vi "Eyecat_Omega_v01.vi"() -> ()   [LabVIEW 2014]
doc: "This VI is an upgrade from the WIN 1_v4 that implements the ageing subrutine"
uses:
  <vilib>/Utility/miscctls.llb/LVRowAndColumnTypeDef.ctl
  Buttons/Numeric control.ctl
  Buttons/String input.ctl
  Buttons/Numeric indicator.ctl
  Controls Win/Control 3.ctl
  <vilib>/Platform/TimedLoop/XDataNode/nitl_modes.ctl
  <vilib>/Platform/TimedLoop/XDataNode/timing_clust.ctl
  <vilib>/Platform/TimedLoop/XDataNode/wakeup.ctl
  <vilib>/Utility/miscctls.llb/LVComboBoxStrsAndValuesArrayTypeDef.ctl
  <vilib>/Utility/miscctls.llb/LVPositionTypeDef.ctl
  <vilib>/Utility/miscctls.llb/LVBoundsTypeDef.ctl
  <vilib>/Utility/file.llb/Read From Spreadsheet File (DBL).vi
  <vilib>/Utility/file.llb/Write To Spreadsheet File (string).vi
  <vilib>/Utility/file.llb/Read From Spreadsheet File (string).vi
  <vilib>/Platform/TimedLoop/XDataNode/XDataNode.xnode
  <vilib>/Platform/TimedLoop/XDataNode/XDNodeRunTimeDep.lvlib
panel:
  in  "Column Length":i32=12
  in  "Cycle Directory":string="c:\\Setup Files\\Ageing Cycles\\Omicron"
  in  "Omicron":bool
  out "Loop Number":dbl
  out "Mexa 3 IP":bool
  out "Mexa 2 IP":bool
  out "Mexa 1 IP":bool
  out "SMS":bool
  out "Directory":string
  out "Vehicle Name":string
  out "output cluster":T1
  out "SMS Recipients":u32
  out "Text Alerts":bool
  out "ETAS-D":bool
  out "ETAS Out":dbl[](array[numeric])
  out "MKS 1":dbl[](array[numeric])
  out "Mexa 3":dbl[](array[numeric])
  out "Mexa 2":dbl[](array[numeric])
  out "Mexa 1":dbl[](array[numeric])
  in  "Inlet LAMBDA Lean":T2=1.2 min=1.02 max=3.0 step=0.001
  in  "NO ppm SW":dbl=500.0 caption="NO (ppm)" min=0.0 max=500.0 step=1.0
  in  "Inlet Temperature (°C)":T2=400.0 min=350.0 max=1000.0 step=1.0
  out "File Directory":string
  out "OFF":bool
  out "COOL":bool
  out "TEST":bool
  out "WMUP":bool
  out "STBY":bool
  out "Mexa-3":bool
  out "Mexa-2":bool
  out "Mexa-1":bool
  out "Heat Load Control":bool
  out "Cycle Length":dbl
  out "Time Remaining":dbl=30.0 format="%<%H:%M:%S>t"
  out "Analysers":u32
  out "% Complete":u8(slide) scale=0.0..100.0
  out "Log?":bool
  in  "Total Number of Cycles":T2=1.0 min=1.0 max=10000.0 step=1.0
  in  "Sub-Cycle Pattern":string[][](table) caption="Subcycle pattern"
  in  "Delete Cycle":bool
  in  "Load Cycle":bool
  in  "Cycle Name":T3
  in  "Save Cycle":bool
  in  "Clear Cycle Pattern":bool
  in  "Menu_Tab":enum32{"Page 1"}(tab)
  in  "Back_Menu":bool
  in  "Home 2":bool
  in  "Performance 2":bool
  in  "Ageing 2":bool
  in  "System 2":bool
  in  "MFC 2":bool
  in  "Analyser 2":bool
  in  "Alarm 2":bool
  in  "Menu":bool
  out "MFC Array":dbl[](array[numeric])
  out "Valve Array":dbl[](array[numeric])
  out "MKS":bool
  out "Pressure":dbl
  out "ExtAnDn":bool
  out "ExtAnUp":bool
  out "File name":string
  out "Log interval (seconds)":T2
  in  "Flow rate Age":dbl
  in  "Inlet temp Age":dbl
  out "Stopped?":bool
  in  "Stop Cmd":T2
  out "Connected?":bool
  out "Error":dbl
  out "Iteration Duration":i64
  out "Finished Late? [i-1]":bool
  out "stop 2":bool
  in  "Enum 1":i16=1
  in  "Acknowledge":bool
  out "Test number":u16
  out "Flag1":bool=TRUE
  out "EditPos Subc":T4
  in  "Tab Control":T5(tab)
  in  "Admin":bool
  out "Warm Up":bool
  in  "Leak Test":bool
  in  "Stop Test":bool
  in  "Log Test Data":bool
  in  "Start Test":bool
  in  "Adv Settings":bool
  out "Doors Unlocked":bool
  in  "File Name":T3="Test"
  out "Fail":bool
  out "Pass":bool
  in  "Select Test Type":T6(radio)=enum."Ageing Test"
  out "Standby":bool
  out "Doors Open":bool
  out "Extractor Fan On":bool
  out "Test In Progress":bool
  out "Cool Down":bool
  out "System Alarm":bool
  in  "Nitrogen Injection (l/min)":T2=50.0 min=0.0 max=250.0 step=0.01
  in  "Oxidation Duration (min)":T2=1.0 min=0.0 max=60.0 step=0.01
  in  "Oxidation Wait (min)":T2=5.0 min=0.0 max=60.0 step=0.001
  in  "Reduction Duration (min)":T2=1.0 min=0.0 max=60.0 step=0.001
  in  "Reduction Wait (min)":T2=7.0 min=0.0 max=60.0 step=0.01
  out "OSC Results":string[][](table) caption="Subcycle pattern"
  in  "Test Stop temperature (°C)":T2=300.0 min=100.0 max=1000.0 step=1.0
  in  "Test Start Temperature (°C)":T2=125.0 min=0.0 max=500.0 step=1.0
  in  "Furnace Ramp Rate (°C/min)":T2=15.0 min=1.0 max=50.0 step=0.1
  in  "NO:CO Ratio":T2=1.1 min=1.0 max=5.0 step=0.1
  in  "Inlet O2 (%)":T2=0.5 min=0.0 max=14.0 step=0.01
  in  "Inlet LAMBDA":T2=1.0 min=0.6 max=3.0 step=0.001
  out "Space Velocity (h-1)":T7
  out "Vol Flow @ STP (l/min)":T7
  in  "Test Flow Rate(g/s)":T2 min=0.0 max=100.0 step=0.01
  out "Sample Volume (litres)":T7
  in  "Number of Samples":T2=1.0 min=1.0 max=6.0 step=1.0
  in  "Sample Diameter (mm)":T2
  out "CO Theory (%) NO":T7 format="%#_3g"
  out "CO Theory (%)":T7 format="%#_3g"
  out "HC Theory (%)":T7
  in  "Sample Length (mm)":T2 min=0.0 step=0.5
  in  "NO ppm Loff":T2 caption="NO ppm"
  in  "Ageing - Cycle Pattern":string[][](table) caption="Subcycle pattern"
  in  "Export Cycle":bool
  in  "Graph Cycle Box 2":string(combo)="CO"
  out "MFC Graph 6":dynamicdata(graph)
  in  "Graph Cycle Box":string(combo)="CO"
  in  "Compile Test Button 2":bool
  in  "Import Data":bool
  in  "Delete sCycle":bool
  in  "Save sCycle":bool
  in  "Load sCycle":bool
  in  "Clear subcycle":bool
  out "MFC Graph 5":dynamicdata(graph)
  out "Test Compiled":bool
  in  "Cycle List":i32(listbox)=1
  in  "Cycle Name":T3
  out "Heat Exchanger Temperatures (°C)":dynamicdata(graph)
  out "System Pressure (kPa)":dynamicdata(graph)
  out "Flow 2":dbl=30.0 format="%#.2g"
  out "Flow 1":dbl=30.0 format="%#.2g"
  out "TC 2":dbl=30.0 format="%#.3g"
  out "TC 6":dbl=30.0 format="%#.3g"
  out "TC 5":dbl=30.0 format="%#.3g"
  out "TC 4":dbl=30.0 format="%#.3g"
  out "TC 3":dbl=30.0 format="%#.3g"
  out "TC 1":dbl=30.0 format="%#.3g"
  out "Gas Flow Measurement Temperatures (°C)":dynamicdata(graph)
  out "Flow Rate (g/s)":dynamicdata(graph)
  out "Sample Temperatures (°C)":dynamicdata(graph)
  out "System Temperatures (°C)":dynamicdata(graph)
  in  "Graph 6 Box":string(combo)="NO"
  in  "Graph 5 Box":string(combo)="HC Cycle 1"
  out "MFC Graph 6":dynamicdata(graph)
  out "MFC Graph 5":dynamicdata(graph)
  in  "Graph 1 Box":string(combo)="CO"
  in  "Graph 4 Box":string(combo)="NO"
  in  "Graph 3 Box":string(combo)="Air Cycle 1"
  in  "Graph 2 Box":string(combo)="HC Cycle 1"
  out "MFC Graph 4":dynamicdata(graph)
  out "MFC Graph 3":dynamicdata(graph)
  out "MFC Graph 1":dynamicdata(graph)
  out "MFC Graph 2":dynamicdata(graph)
  out "CO2 Concentration (%)":dynamicdata(graph)
  out "Lambda":dynamicdata(graph)
  out "HC Concentration (ppm)":dynamicdata(graph)
  out "O2 Concentration (%)":dynamicdata(graph)
  out "CO Concentration (%)":dynamicdata(graph)
  out "NO Concentration (ppm)":dynamicdata(graph)
  in  "Purge System":bool
  in  "Alarm ack":bool
  in  "Clear log":bool
  out "Table":string[][](table)
  out "Soft Alarm":bool
  out "Hard Alarm":bool
  # "0.96 < lambda < 0.85"
  # "1.02< lambda < 1.6"
  # "350 < Tinlet < 1000"
  # "Test Commands"
  # "System Indicators"
  # "Test Type"
  # "Leak Test"
  # "Lightoff Settings"
  # "Catalyst Specification"
  # "Furnace Lightoff Settings"
  # "OSC Settings"
  # "CO/HC Lightoff Settings"
  # "Flow Specification"
  # "NO Lightoff Settings"
  # "Cycle Compiled"
  # "°C"
  # "°C"
  # "°C"
  # "°C"
  # "°C"
  # "°C"
  # "g/s"
  # "g/s"
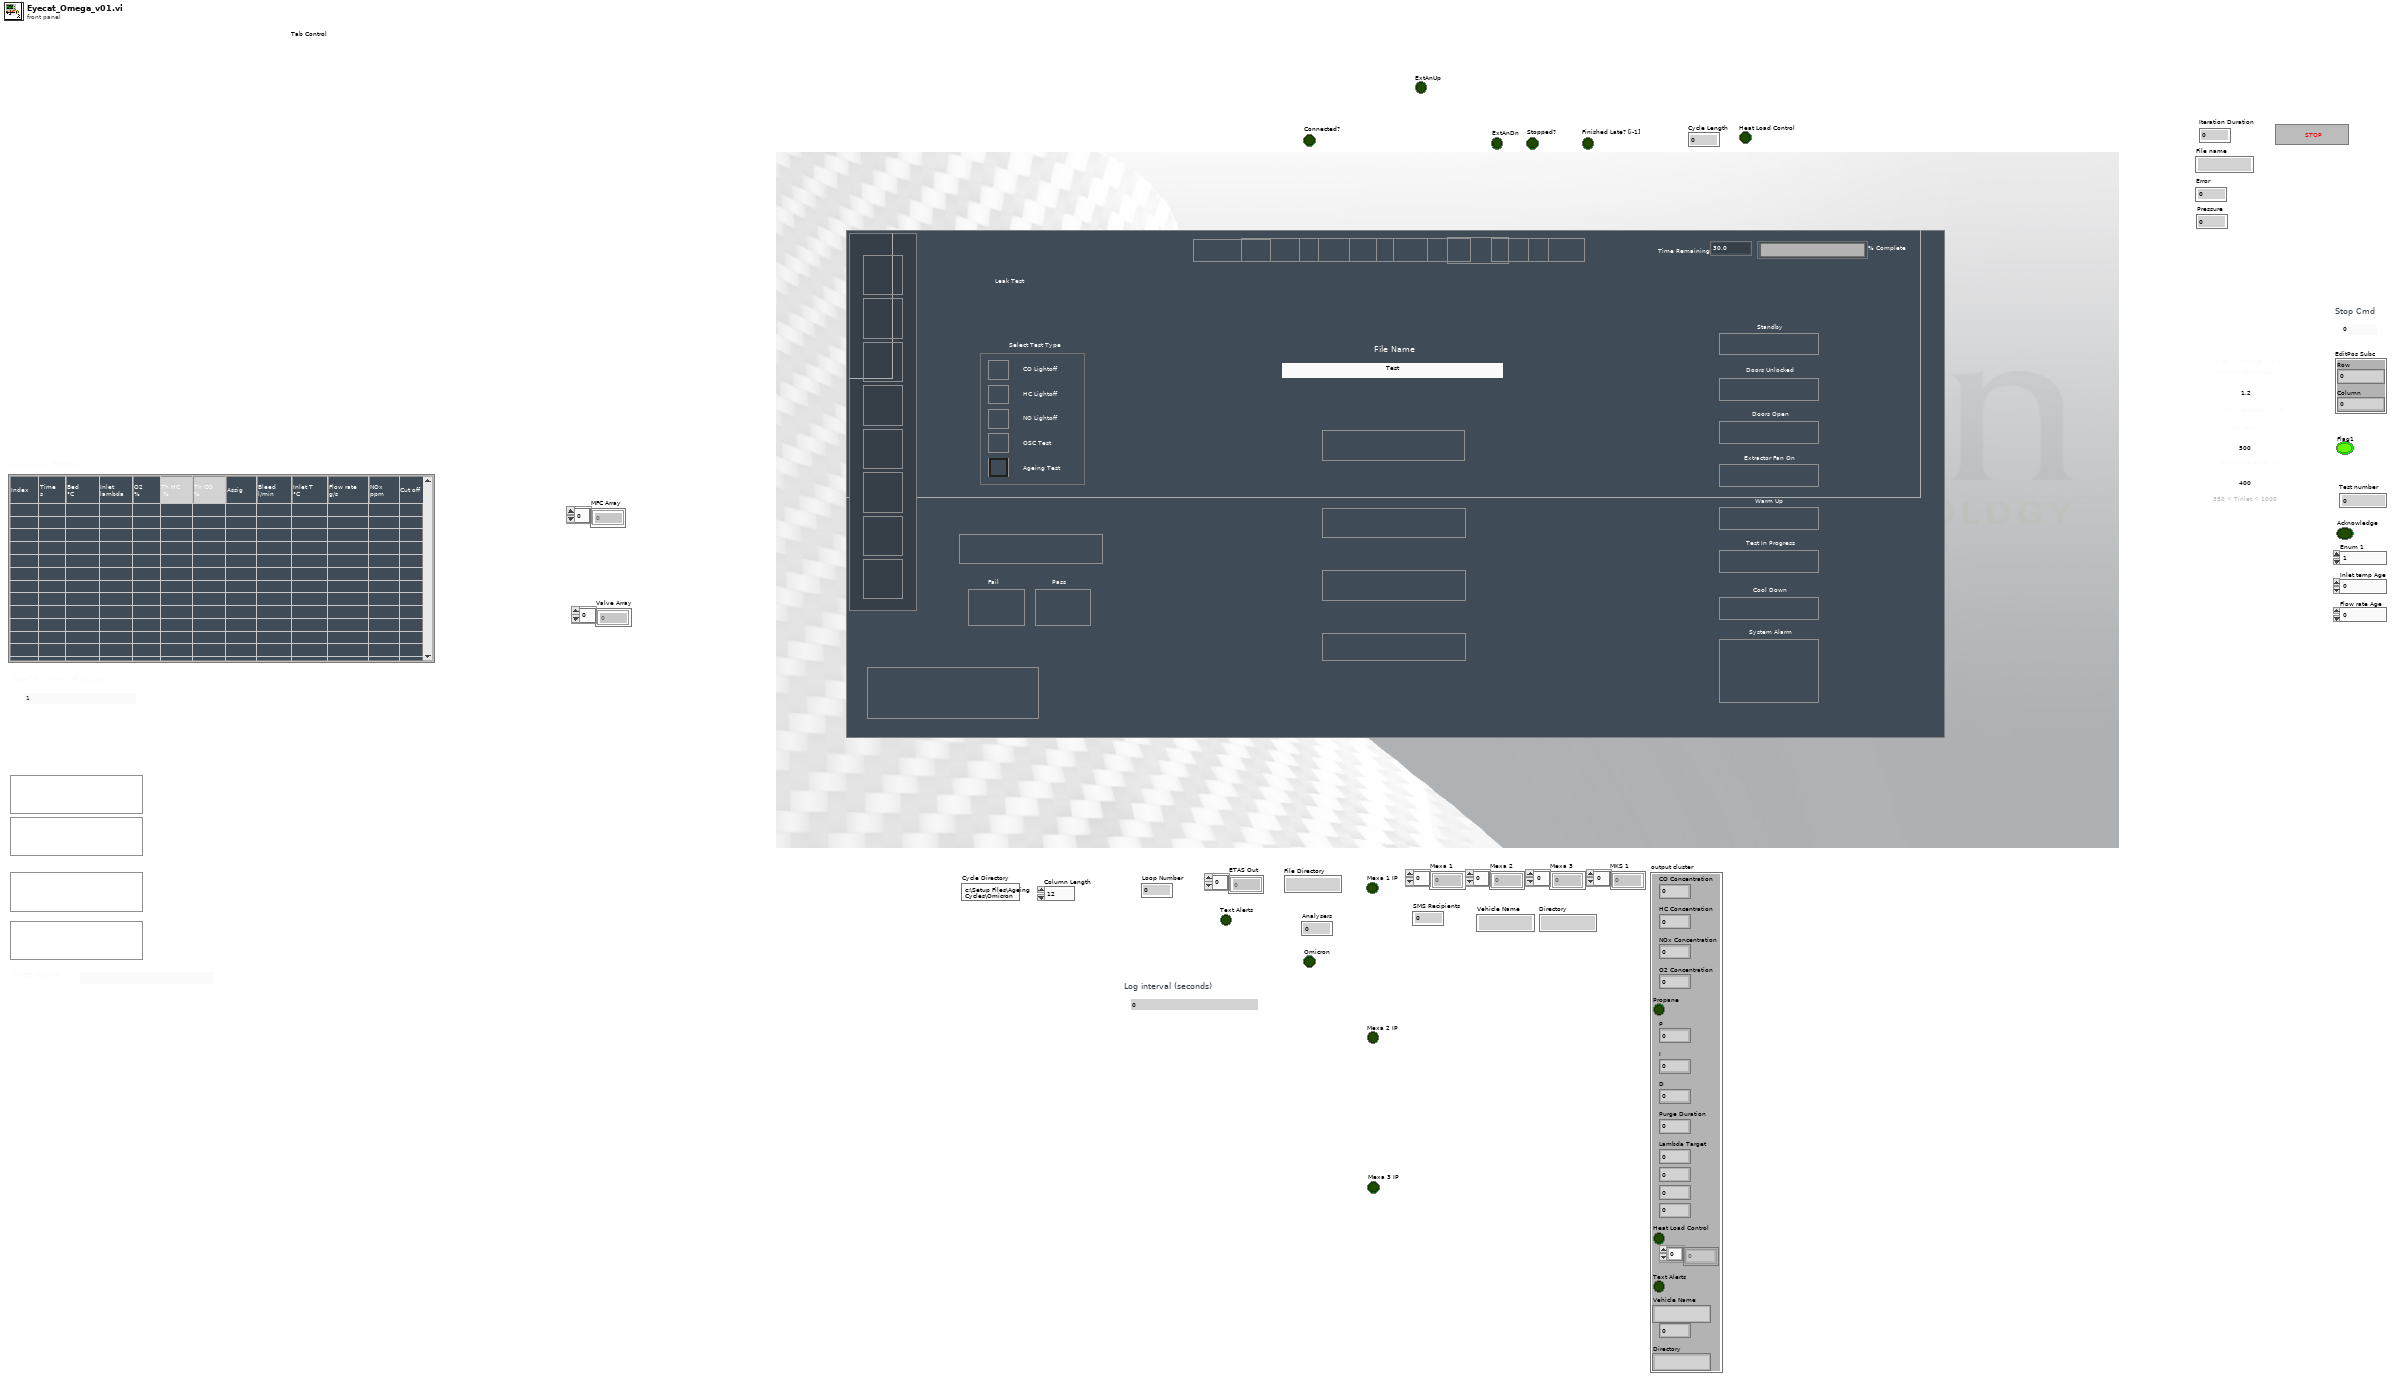
[diagram p1: front panel]
types:
  T1 = cluster{"CO Concentration":dbl, "HC Concentration":dbl, "NOx Concentration":dbl, "O2 Concentration":dbl, "Propane":bool, "P":dbl, "I":dbl, "D":dbl, "Purge Duration":dbl, "Lambda Target":dbl, dbl, u32, dbl, "Heat Load Control":bool, dbl[], "Text Alerts":bool, "Vehicle Name":string, u32, "Directory":string}
  T2 = typedef "Numeric control.ctl" = dbl
  T3 = typedef "String input.ctl" = string
  T4 = typedef "LVRowAndColumnTypeDef.ctl" = cluster{"Row":i32, "Column":i32}
  T5 = enum32{"MAIN", "PERFORMANCE TEST SETUP", "AGEING TEST SETUP", "SCHEDULE", "SYSTEM DATA", "MFC", "ANALYSER DATA", "ALARM LOG"}
  T6 = enum32{"CO Lightoff", "HC Lightoff", "NO Lightoff", "OSC Test", "Ageing Test"}
  T7 = typedef "Numeric indicator.ctl" = dbl
  T8 = typedef "XDNodeRunTimeDep.lvlib/nitl_modes.ctl" = enum32{"No Change", "Process missed periods, maintain original phase", "Discard missed periods, maintain original phase", "Process missed periods, ignore original phase", "Discard missed periods, ignore original phase"}
  T9 = typedef "Control 3.ctl" = enum16{"main", "start test", "save subc", "load subc", "delete subc", "clear table 1", "update list 1", "save cycle", "load cycle", "delete cycle", "clear table 2", "update list 2", "calc HC CO", "Total time calc", "update Cycle pattern ", "load cycle name", "convert to num", "load test array", "check scycle name", "check cycle name", "Multigas connect", "Multigas disconnect", "Leak Test", "Import Cycle", "Display Graph", "Export Cycle"}
  T10 = typedef "LVComboBoxStrsAndValuesArrayTypeDef.ctl" = cluster{"String":string, "Value":string}[]
  T11 = cluster{"CO Concentration":dbl, "CO Concentration":dbl, "CO Concentration":dbl, "CO Concentration":dbl, "Propane":bool, "CO Concentration":dbl, "CO Concentration":dbl, "CO Concentration":dbl, "CO Concentration":dbl, "CO Concentration":dbl, "CO Concentration":dbl, u32, "CO Concentration":dbl, "Propane":bool, dbl[], "Propane":bool, "Vehicle Name":string, u32, "Vehicle Name":string}
  T12 = typedef "XDNodeRunTimeDep.lvlib/timing_clust.ctl" = cluster{"Expected End [f-1]":u64, "Actual End [f-1]":u64, "Finished Late? [f-1]":bool, "Expected End [i-1]":u64, "Actual End [i-1]":u64, "Finished Late? [i-1]":bool, "Expected Start [i]":u64, "Actual Start [i]":u64, "Expected Start [f]":u64, "Actual Start [f]":u64, "Source Name":string, "Structure Name":string, "Period":i64, "Deadline":i64, "Offset":i64, "Start":i64, "Priority":i32, "Timeout":i32, "Mode":T8, "Wakeup Reason":T13, "Error":errorcluster, "Source Type":string, "Secondary Source Type":string, "Global End Time":u64, "Global Start Time":u64, "Frame Duration":u64, "Iteration Duration":u64, "Assigned CPU":i32, "I/O Scan Engine Mode":u32}
  T13 = typedef "XDNodeRunTimeDep.lvlib/wakeup.ctl" = enum32{"Normal", "Aborted", "Asynchronous wakeup", "Timing source error", "Timed loop error", "Timeout"}
  T14 = enum8{"Enabled", "Disabled", "Disabled and Grayed Out"}
  T15 = typedef "LVPositionTypeDef.ctl" = cluster{"Left":i32, "Top":i32}
  T16 = typedef "LVBoundsTypeDef.ctl" = cluster{"Width":u32, "Height":u32}
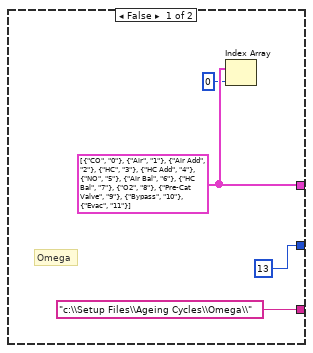
[diagram p2: hidden frame]
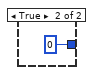
[diagram p4: hidden frame]
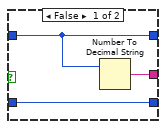
[diagram p5: hidden frame]
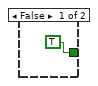
[diagram p7: hidden frame]
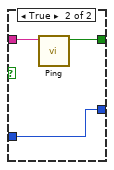
[diagram p9: hidden frame]
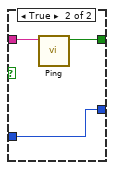
[diagram p11: hidden frame]
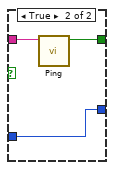
[diagram p13: hidden frame]
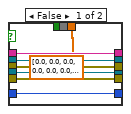
[diagram p15: hidden frame]
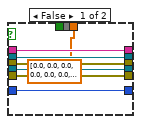
[diagram p16: hidden frame]
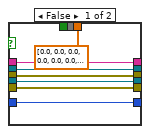
[diagram p17: hidden frame]
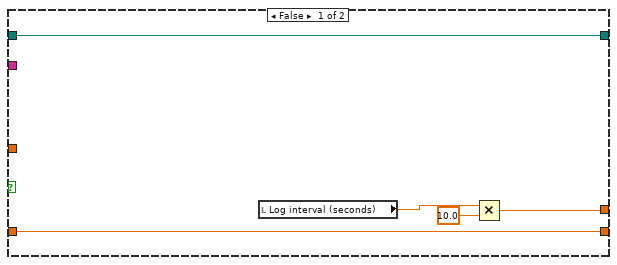
[diagram p18: hidden frame]
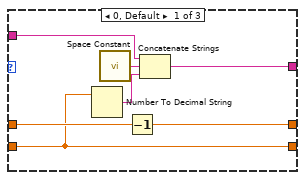
[diagram p19: hidden frame]
diagram:
  w1 = "6" ("Graph Cycle Box")
  w18 = u16 0 ("Test number")
  w40 = "" ("Vehicle Name")
  w39 = u32 0
  w41 = FALSE ("Propane")
  w42 = 0.0 ("CO Concentration")
  w44 = 0.0 ("Numeric")
  w30 = i64 50 ("Period")
  w13 = "C:\\Setup Files\\" ("string")
  (unwired) 12 ("length")
  w67 = FALSE ("Visible")
  w50 = i64 100 ("Period")
  w68 = FALSE
  w72 = FALSE
  w47 = 0.0 ("y")
  w84 = ""
  w89 = u32 13816530
  # "Menu Tabs"
  # "Initial Conditions"
  # "Ageing Table\nColumn No"
  # "0   Flow Rate 1\n1   Flow Rate 2\n     ECM 1\n     ECM 2\n2   CO2 U\n3   CO U\n4   HC U\n5   O2 U\n7   CO2 D\n8   CO D\n9   HC D\n10 O2 D\n12 TC1X\n13 TC2A\n14 TC3Y\n15 TC4B\n16 TC5\n17 TC6\n32 Venturi 1\n33 Venturi 2\n34 Tank\n35 Bearing 1\n36 Bearing 2\n38 Ex A\n39 Ex B\n40 Ex C\n41 Ex D\n     MFC Box\n42 Furnace 1\n43 Furnace 2\n44 NO 1 ?? \n45 Lambda 1\n46 NO 2 ??\n47 Lambda 2\n56 CO (L)\n57 CO (H)\n58CO2\n59 O2\n60 THC\n61 NO\n62 NOx\n63 NO2"
  # "~~~~~~~~~~~~~\n    Data Log Array\n~~~~~~~~~~~~~\n00 Status Integer\n01 Zero Constant\n\n02 DI no1 -errors\n03 DI no2 -states\n04 Flow rate 1 g/s\n05 Flow rate 2 g/s\n06 ECM 1 AFR\n07 ECM 2 AFR\n~~~~~~~~~~~~~\n     Mexa 518 - 1\n~~~~~~~~~~~~~\n08 CO2 %\n09 CO   %\n10 HC   ppm\n11 O2   %\n12 NOx ppm\n~~~~~~~~~~~~~\n     Mexa 518 - 2\n~~~~~~~~~~~~~\n13 CO2 %\n14 CO   %\n15 HC   ppm\n16 O2   %\n17 NOx ppm\n~~~~~~~~~~~~~\n     Temp Array I\n~~~~~~~~~~~~~\n18 1\n19 2 \n20 3\n21 4\n22 5\n23 6\n24 7\n25 8\n26 9\n27 10\n28 11\n29 12\n30 13\n31 14\n32 15\n33 16\n~~~~~~~~~~~~~\n     Temp Array II\n~~~~~~~~~~~~~\n34 17\n35 18\n36 19\n37 20\n38 Vent 1\n39 Vent 2\n40 Tank\n41 Bearing 1\n42 Bearing 2\n43 Cabinet\n44 Ex A\n45 Ex B\n46 Ex C\n47 Ex D\n48 Spare\n~~~~~~~~~~~~~\n49 Furnace Temp 1\n50 Furnace Temp 2\n51 Tank Pressure\n52 Rapidox\n~~~~~~~~~~~~~\n53 NOx L1\n54 NOx L2\n55 NOx 1\n56 NOx 2\n57 UEGO 1\n58 UEGO 2\n59 Switch Valve\n60 UEGO 3\n61 UEGO 4\n\n62 Teff\n\n63 Fan 1 Speed V\n64 Fan 2 Speed V"
  n1 = Concatenate Strings(w13, "Admin" ("string")) -> (w15:string)
  n2 = String To Path(string=w15) -> (path=w14:path)
  n3 = call-poly <vilib>:"Read From Spreadsheet File.vi"("file path (dialog if empty)"=w14) -> ("first row"=w9:dbl[])  [unwired: 6 in, 4 out]
  n4 = Index Array(array=w9, index=15) -> (element=w10:dbl)
  n5 = Number To Boolean Array(number=w10) -> (Boolean array=w12:bool[])
  n6 = Index Array(array=w12, index=2) -> (element=w7:bool)
  n7 = case shown="True" w7 {
    tunnel: ["c:\\Setup Files\\Ageing Cycles\\Omega\\" "c:\\Setup Files\\Ageing Cycles\\Omicron\\"] -> w5
    tunnel: [13 ("length") 20 ("length")] -> w2
    tunnel: [w96 T10 [{"String"="CO-1", "Value"="0"}, {"String"="Air-1", "Value"="1"}, {"String"="Air-1 Add", "Value"="2"}, {"String"="HC-1", "Value"="3"}, {"String"="HC-1 Add", "Value"="4"}, {"String"="O2-1", "Value"="5"}, {"String"="CO-2", "Value"="6"}, {"String"="Air-2", "Value"="7"}, {"String"="Air-2 Add", "Value"="8"}, {"String"="HC-2", "Value"="9"}, {"String"="HC-2 Add", "Value"="10"}, {"String"="O2-2", "Value"="11"}, {"String"="Air Bal", "Value"="12"}, {"String"="HC Bal", "Value"="13"}, {"String"="Cat-1 Valve", "Value"="14"}, {"String"="Cat-2 Valve", "Value"="15"}, {"String"="Bypass Valve", "Value"="16"}, {"String"="Evac-1", "Value"="17"}, {"String"="Evac-2", "Value"="18"}] ("Strings And Values []")] -> w4
    frame False {
      w96 = T10 [{"String"="CO", "Value"="0"}, {"String"="Air", "Value"="1"}, {"String"="Air Add", "Value"="2"}, {"String"="HC", "Value"="3"}, {"String"="HC Add", "Value"="4"}, {"String"="NO", "Value"="5"}, {"String"="Air Bal", "Value"="6"}, {"String"="HC Bal", "Value"="7"}, {"String"="O2", "Value"="8"}, {"String"="Pre-Cat Valve", "Value"="9"}, {"String"="Bypass", "Value"="10"}, {"String"="Evac", "Value"="11"}] ("Strings And Values []")
      # "Omega"
      n8 = Index Array(array=w96, index=0) -> ()  [unwired: 1 out]
    }
    frame True {
      # "Omicron"
    }
  }
  n9 = local write "Cycle Name"(w84) -> ()
  n10 = local write "Cycle Name"(w84) -> ()
  n11 = local write "Test Compiled"(FALSE ("Cycle Compiled")) -> ()
  n12 = local write "Flag1"(FALSE) -> ()
  n13 = local write "Analysers"(u32 0 ("Analysers")) -> ()
  n14 = local write "Sub-Cycle Pattern"(string[][] [["", "0", "", "", "", "", "", "", "", "", "", "", ""], ["", "", "", "", "", "", "", "", "", "", "", "", ""], ["", "", "", "", "", "", "", "", "", "", "", "", ""], ["", "", "", "", "", "", "", "", "", "", "", "", ""], ["", "", "", "", "", "", "", "", "", "", "", "", ""], ["", "", "", "", "", "", "", "", "", "", "", "", ""], ["", "", "", "", "", "", "", "", "", "", "", "", ""], ["", "", "", "", "", "", "", "", "", "", "", "", ""], ["", "", "", "", "", "", "", "", "", "", "", "", ""], ["", "", "", "", "", "", "", "", "", "", "", "", ""], ["", "", "", "", "", "", "", "", "", "", "", "", ""], ["", "", "", "", "", "", "", "", "", "", "", "", ""], ["", "", "", "", "", "", "", "", "", "", "", "", ""], ["", "", "", "", "", "", "", "", "", "", "", "", ""], ["", "", "", "", "", "", "", "", "", "", "", "", ""], ["", "", "", "", "", "", "", "", "", "", "", "", ""], ["", "", "", "", "", "", "", "", "", "", "", "", ""], ["", "", "", "", "", "", "", "", "", "", "", "", ""], ["", "", "", "", "", "", "", "", "", "", "", "", ""], ["", "", "", "", "", "", "", "", "", "", "", "", ""], ["", "", "", "", "", "", "", "", "", "", "", "", ""], ["", "", "", "", "", "", "", "", "", "", "", "", ""], ["", "", "", "", "", "", "", "", "", "", "", "", ""], ["", "", "", "", "", "", "", "", "", "", "", "", ""], ["", "", "", "", "", "", "", "", "", "", "", "", ""], ["", "", "", "", "", "", "", "", "", "", "", "", ""], ["", "", "", "", "", "", "", "", "", "", "", "", ""], ["", "", "", "", "", "", "", "", "", "", "", "", ""], ["", "", "", "", "", "", "", "", "", "", "", "", ""], ["", "", "", "", "", "", "", "", "", "", "", "", ""], ["", "", "", "", "", "", "", "", "", "", "", "", ""]]) -> ()
  n15 = shared-variable "RT CompactRIO Target\\Library 1.lvlib\\Enum 1"(u16 0 ("Enum 1")) -> ()  [unwired: 1 in, 1 out]
  n16 = property on="Tab Control" class="TabCtl (strict)"("Value"=T5."MAIN" ("Tab Control")) -> ()  [unwired: 2 in, 2 out]
  n17 = Bundle("CO Concentration"=w42, "CO Concentration"=w42, "CO Concentration"=w42, "CO Concentration"=w42, "Propane"=w41, "CO Concentration"=w42, "CO Concentration"=w42, "CO Concentration"=w42, "CO Concentration"=w42, "CO Concentration"=w42, "CO Concentration"=w42, w39, "CO Concentration"=w42, "Propane"=w41, dbl[] [0.0, 0.0, 0.0, 2.0, 1.0], "Propane"=w41, "Vehicle Name"=w40, w39, "Vehicle Name"=w40) -> (w43:T11)  [unwired: 1 in]
  n18 = local write "output cluster"(w43) -> ()
  n19 = property on="Sub-Cycle Pattern" class="Tbl (strict)"("Active Cell"=T4 {"Row"=-2, "Column"=5} ("Active Cell:Active Cell"), "Cell BG Color"=w89) -> (error out=w90:errorcluster)  [unwired: 2 in, 1 out]
  n20 = property on="Sub-Cycle Pattern" class="Tbl (strict)"(error in=w90, "Active Cell"=T4 {"Row"=-2, "Column"=6} ("Active Cell:Active Cell"), "Cell BG Color"=w89) -> ()  [unwired: 1 in, 2 out]
  n21 = local write "Fail"(w72) -> ()
  n22 = local write "Pass"(w72) -> ()
  n23 = property on="Pass" class="Bool (strict)"("Value"=w72) -> ()  [unwired: 2 in, 2 out]
  n24 = property on="Fail" class="Bool (strict)"("Value"=w72) -> ()  [unwired: 2 in, 2 out]
  n25 = property on="System Alarm" class="Bool (strict)"("Value"=w72) -> ()  [unwired: 2 in, 2 out]
  n26 = property on="Soft Alarm" class="Bool (strict)"("Value"=w72) -> ()  [unwired: 2 in, 2 out]
  n27 = property on="Hard Alarm" class="Bool (strict)"("Value"=w72) -> ()  [unwired: 2 in, 2 out]
  n28 = property on="TEST" class="Bool (strict)"("Visible"=w67) -> ()  [unwired: 2 in, 2 out]
  n29 = property on="OFF" class="Bool (strict)"("Visible"=w67) -> ()  [unwired: 2 in, 2 out]
  n30 = property on="WMUP" class="Bool (strict)"("Visible"=w67) -> ()  [unwired: 2 in, 2 out]
  n31 = property on="STBY" class="Bool (strict)"("Visible"=w67) -> ()  [unwired: 2 in, 2 out]
  n32 = property on="COOL" class="Bool (strict)"("Visible"=w67) -> ()  [unwired: 2 in, 2 out]
  n33 = local write "Connected?"(w72) -> ()
  n34 = local write "Acknowledge"(w72) -> ()
  n35 = String To Path(string="c:\\Setup Files\\Cycles Folder\\") -> (path=w86:path)
  n36 = String To Path(string=w5) -> (path=w87:path)
  n37 = List Folder(path=w86, pattern="*.eyec") -> ()  [unwired: 2 in, 4 out]
  n38 = List Folder(path=w87, pattern="*.eyes") -> (filenames=w88:string[])  [unwired: 2 in, 3 out]
  n39 = Obtain Queue(element data type=Control_3."main" ("Enum")) -> (queue out=w93:refnum<queue>)  [unwired: 4 in, 2 out]
  n40 = property on="Cycle Directory" class="Str"("Value"=w5) -> ()  [unwired: 2 in, 2 out]
  n41 = Decrement(x=w2) -> (x-1=w3:i32)
  n42 = property on="Graph Cycle Box" class="CmbBox"("Strings And Values[]"=w4, "Value"=w1) -> ()  [unwired: 2 in, 2 out]
  n43 = property on="Graph Cycle Box 2" class="CmbBox"("Strings And Values[]"=w4, "Value"=w1) -> ()  [unwired: 2 in, 2 out]
  n44 = property on="Cycle List" class="LstBox (strict)"("Item Names"=w88) -> ()  [unwired: 2 in, 2 out]
  n45 = local write "Mexa 1 IP"(FALSE ("Mexa 1 IP")) -> ()
  n46 = property on="Column Length" class="DigNum (strict)"("Value"=w3) -> ()  [unwired: 2 in, 2 out]
  n47 = Concatenate Strings(w13, "Admin" ("string")) -> (w64:string)
  n48 = Concatenate Strings(w13, "Admin IP" ("string")) -> (w63:string)
  n49 = String To Path(string=w63) -> (path=w31:path)
  n50 = String To Path(string=w64) -> (path=w61:path)
  n51 = node-c288(w50) -> (w60:T12)  [unwired: 3 in]
  n52 = node-c288(w50) -> (w58:T12)  [unwired: 3 in]
  n53 = node-c288(w50) -> (w56:T12)  [unwired: 3 in]
  n54 = node-c288() -> (w54:T12)  [unwired: 4 in]
  n55 = node-c288(w50) -> (w52:T12)  [unwired: 3 in]
  n56 = timed-loop {
    timing: w60 -> [_]
    timing-out: [_] -> w59
    shift-right: [w116] -> _
    shift-left: _ -> [w115]
    shift-right: [w113] -> _
    shift-left: _ -> [w109]
    shift-right: [w114] -> _
    shift-left: _ -> [w110]
    shift-right: [w112] -> _
    shift-left: _ -> [w108]
    shift-right: [w111] -> _
    shift-left: _ -> [w107]
    shift-right: [w106] -> _
    shift-left: _ -> [w105]
    tunnel: w31 -> [w103]
    stop <- _ stop-if-true
    n57 = node-c288() -> ()  [unwired: 1 in, 1 out]
    n58 = call-poly <vilib>:"Read From Spreadsheet File.vi"("file path (dialog if empty)"=w103) -> ("first row"=w123:string[])  [unwired: 6 in, 4 out]
    n59 = local read "Analysers"() -> (w120:u32)
    n60 = Array Subset(array=w123, index=0 ("length"), length=2) -> (w121:string[])
    n61 = Number To Boolean Array(number=w120) -> (Boolean array=w119:bool[])
    n62 = local read "Mexa 1 IP"() -> (w102:bool)
    n63 = Index Array(array=w119, index=0) -> (element=w117:bool)
    "Mexa-1" <- w117
    n64 = case shown="True" w102 {
      tunnel: w121 -> [_ w146]
      tunnel: w117 -> [_ w145]
      tunnel: [w131 w144] -> w116
      tunnel: w115 -> [w131 w143]
      tunnel: [w130 w142] -> w114
      tunnel: [w129 w141] -> w113
      tunnel: [w128 w140] -> w112
      tunnel: [w127 w139] -> w111
      tunnel: w110 -> [w130 w138]
      tunnel: w109 -> [w129 w137]
      tunnel: w108 -> [w128 w136]
      tunnel: w107 -> [w127 w135]
      tunnel: [w126 w134] -> w106
      tunnel: w105 -> [w126 w133]
      tunnel: [dbl[] [0.0, 0.0, 0.0, 0.0, 0.0, 0.0, 0.0] ("Emissions") w132] -> w104
      frame False {
      }
      frame True {
        n65 = call "Mexa_7170.vi"("String 1 In"=w143, "Connect"=w145, "IP Array"=w146, "connection ID 1 In"=w138, "error out 1 In"=w137, "connection ID 2 In"=w136, "error out 2 In"=w135, "Time In"=w133) -> ("Emissions"=w132:dbl[], "String 1 Out"=w144:string, "connection ID 1 Out"=w142:refnum<k5>, "error 1 out"=w141:errorcluster, "connection ID 2 Out"=w140:refnum<k16>, "Time Out"=w134:i16, "error 2 out"=w139:errorcluster)  [unwired: 1 in]
      }
    }
    "Mexa 1" <- w104
    n66 = node-c288() -> ()  [unwired: 1 in, 1 out]
  }
  n67 = timed-loop {
    timing: w58 -> [_]
    timing-out: [_] -> w57
    shift-right: [w163] -> _
    shift-left: _ -> [w164]
    shift-right: [w161] -> _
    shift-left: _ -> [w157]
    shift-right: [w162] -> _
    shift-left: _ -> [w158]
    shift-right: [w160] -> _
    shift-left: _ -> [w156]
    shift-right: [w159] -> _
    shift-left: _ -> [w155]
    shift-right: [w153] -> _
    shift-left: _ -> [w154]
    tunnel: w31 -> [w166]
    stop <- _ stop-if-true
    n68 = node-c288() -> ()  [unwired: 1 in, 1 out]
    n69 = call-poly <vilib>:"Read From Spreadsheet File.vi"("file path (dialog if empty)"=w166) -> ("first row"=w171:string[])  [unwired: 6 in, 4 out]
    n70 = local read "Analysers"() -> (w169:u32)
    n71 = Array Subset(array=w171, index=2 ("length"), length=2) -> (w165:string[])
    n72 = Number To Boolean Array(number=w169) -> (Boolean array=w168:bool[])
    n73 = local read "Mexa 2 IP"() -> (w149:bool)
    n74 = Index Array(array=w168, index=1) -> (element=w152:bool)
    "Mexa-2" <- w152
    n75 = case shown="True" w149 {
      tunnel: w165 -> [_ w194]
      tunnel: w164 -> [w179 w193]
      tunnel: [w179 w192] -> w163
      tunnel: [w178 w191] -> w162
      tunnel: [w177 w190] -> w161
      tunnel: [w176 w189] -> w160
      tunnel: [w175 w188] -> w159
      tunnel: w158 -> [w178 w187]
      tunnel: w157 -> [w177 w186]
      tunnel: w156 -> [w176 w185]
      tunnel: w155 -> [w175 w184]
      tunnel: w154 -> [w174 w183]
      tunnel: [w174 w182] -> w153
      tunnel: w152 -> [_ w181]
      tunnel: [dbl[] [0.0, 0.0, 0.0, 0.0, 0.0, 0.0, 0.0] ("Emissions") w180] -> w151
      frame False {
      }
      frame True {
        n76 = call "Mexa_7170 - 2.vi"("String 1 In"=w193, "Connect"=w181, "IP Array"=w194, "connection ID 1 In"=w187, "error out 1 In"=w186, "connection ID 2 In"=w185, "error out 2 In"=w184, "Time In"=w183) -> ("Emissions"=w180:dbl[], "String 1 Out"=w192:string, "connection ID 1 Out"=w191:refnum<k5>, "error 1 out"=w190:errorcluster, "connection ID 2 Out"=w189:refnum<k16>, "Time Out"=w182:i16, "error 2 out"=w188:errorcluster)  [unwired: 1 in]
      }
    }
    n77 = call "7000string to array.vi"("7170 Input"=w151) -> ("7000 Out"=→"Mexa 2":dbl[])  [unwired: 4 in]
    n78 = node-c288() -> ()  [unwired: 1 in, 1 out]
  }
  n79 = timed-loop {
    timing: w56 -> [_]
    timing-out: [_] -> w55
    shift-right: [w211] -> _
    shift-left: _ -> [w212]
    shift-right: [w207] -> _
    shift-left: _ -> [w204]
    shift-right: [w210] -> _
    shift-left: _ -> [w205]
    shift-right: [w209] -> _
    shift-left: _ -> [w203]
    shift-right: [w208] -> _
    shift-left: _ -> [w202]
    shift-right: [w206] -> _
    shift-left: _ -> [w201]
    tunnel: w31 -> [w214]
    stop <- _ stop-if-true
    n80 = node-c288() -> ()  [unwired: 1 in, 1 out]
    n81 = call-poly <vilib>:"Read From Spreadsheet File.vi"("file path (dialog if empty)"=w214) -> ("first row"=w219:string[])  [unwired: 6 in, 4 out]
    n82 = local read "Analysers"() -> (w217:u32)
    n83 = Array Subset(array=w219, index=4 ("length"), length=2) -> (w199:string[])
    n84 = Number To Boolean Array(number=w217) -> (Boolean array=w216:bool[])
    n85 = local read "Mexa 3 IP"() -> (w197:bool)
    n86 = Index Array(array=w216, index=2) -> (element=w200:bool)
    "Mexa-3" <- w200
    n87 = case shown="True" w197 {
      tunnel: w212 -> [w227 w242]
      tunnel: [w227 w241] -> w211
      tunnel: [w226 w240] -> w210
      tunnel: [w224 w239] -> w209
      tunnel: [w223 w238] -> w208
      tunnel: [w225 w237] -> w207
      tunnel: [w222 w236] -> w206
      tunnel: w205 -> [w226 w235]
      tunnel: w204 -> [w225 w234]
      tunnel: w203 -> [w224 w233]
      tunnel: w202 -> [w223 w232]
      tunnel: w201 -> [w222 w231]
      tunnel: w200 -> [_ w230]
      tunnel: w199 -> [_ w229]
      tunnel: [dbl[] [0.0, 0.0, 0.0, 0.0, 0.0, 0.0, 0.0] ("Emissions") w228] -> w198
      frame False {
      }
      frame True {
        n88 = call "Mexa_7170 - 3.vi"("String 1 In"=w242, "Connect"=w230, "IP Array"=w229, "connection ID 1 In"=w235, "error out 1 In"=w234, "connection ID 2 In"=w233, "error out 2 In"=w232, "Time In"=w231) -> ("Emissions"=w228:dbl[], "String 1 Out"=w241:string, "connection ID 1 Out"=w240:refnum<k5>, "error 1 out"=w237:errorcluster, "connection ID 2 Out"=w239:refnum<k16>, "Time Out"=w236:i16, "error 2 out"=w238:errorcluster)  [unwired: 1 in]
      }
    }
    n89 = call "7000string to array.vi"("7170 Input"=w198) -> ("7000 Out"=→"Mexa 3":dbl[])  [unwired: 4 in]
    n90 = node-c288() -> ()  [unwired: 1 in, 1 out]
  }
  n91 = timed-loop {
    timing: w54 -> [_]
    timing-out: [_] -> w53
    tunnel: w31 -> [w248]
    stop <- _ stop-if-true
    n92 = node-c288() -> ()  [unwired: 1 in, 1 out]
    n93 = call-poly <vilib>:"Read From Spreadsheet File.vi"("file path (dialog if empty)"=w248) -> ("first row"=w253:string[])  [unwired: 6 in, 4 out]
    n94 = local read "Analysers"() -> (w251:u32)
    n95 = Array Subset(array=w253, index=6 ("length"), length=2) -> (w247:string[])
    n96 = Number To Boolean Array(number=w251) -> (Boolean array=w250:bool[])
    n97 = Index Array(array=w250, index=3) -> (element=w246:bool)
    "MKS" <- w246
    n98 = call "MKS.vi"("IP Array"=w247, "Connect"=w246) -> ("Emissions"=→"MKS 1":dbl[])  [unwired: 9 in]
    n99 = node-c288() -> ()  [unwired: 1 in, 1 out]
  }
  n100 = timed-loop {
    timing: w52 -> [_]
    timing-out: [_] -> w51
    tunnel: w31 -> [w275]
    shift-right: [w274] -> _
    shift-left: _ -> [w270]
    shift-right: [w273] -> _
    shift-left: _ -> [w269]
    shift-right: [w272] -> _
    shift-left: _ -> [w268]
    shift-right: [w271] -> _
    shift-left: _ -> [w267]
    shift-right: [w259] -> _
    shift-left: _ -> [w257]
    stop <- _ stop-if-true
    n101 = node-c288() -> ()  [unwired: 1 in, 1 out]
    n102 = call-poly <vilib>:"Read From Spreadsheet File.vi"("file path (dialog if empty)"=w275) -> ("first row"=w280:string[])  [unwired: 6 in, 4 out]
    n103 = local read "Analysers"() -> (w278:u32)
    n104 = Number To Boolean Array(number=w278) -> (Boolean array=w277:bool[])
    n105 = Index Array(array=w280, index=8 ("length")) -> (element=w261:string)
    n106 = Index Array(array=w277, index=4) -> (element=w260:bool)
    "ETAS-D" <- w260
    n107 = call "ETAS_Driver_1.0.2.vi"("Counter In"=w267, "IP Address"=w261, "Loop In"=w268, "error In"=w269, "Reference In"=w270, "Etas Connect"=w260) -> ("Loop Out"=w272:i32, "error out"=w273:errorcluster, "Reference Out"=w274:refnum<k24>, "ETAS Out"=w258:dbl[], "Counter Out"=w271:dbl)  [unwired: 1 in]
    n108 = Index Array(array=w258) -> (element #1=w264:dbl, element #2=w263:dbl)  [unwired: 2 in]
    n109 = Equal To 0?(x=w264) -> (x = 0?=w266:bool)
    n110 = Equal To 0?(x=w263) -> (x = 0?=w265:bool)
    n111 = Compound Arithmetic op=AND(w266, w265, w260) -> (w262:bool)
    n112 = case shown="True" w262 {
      tunnel: [w281 w282] -> w259
      tunnel: w257 -> [_ w282]
      tunnel: w258 -> [w281 _]
      frame False {
      }
      frame True {
      }
    }
    "ETAS Out" <- w259
    n113 = node-c288() -> ()  [unwired: 1 in, 1 out]
  }
  n114 = while {
    tunnel: w93 -> [w292]
    tunnel: [FALSE ("stop 2")] -> w78
    tunnel: w61 -> [w289]
    stop <- w293 stop-if-true
    n115 = Concatenate Strings("Cycle Directory", "\\" ("string")) -> (w285:string)
    n116 = Dequeue Element(queue=w292) -> (element=w291:T9)  [unwired: 2 in, 3 out]
    n117 = case shown="\"load test array\"" w291 {
      tunnel: w285 -> [_ _ _ w351 w362 w399 w432 w463 _ _ _ _ _ _ _ _ _ _ _ _ _ _ _ _ _ w729]
      tunnel: w289 -> [w310 _ _ _ _ _ _ _ _ _ _ _ _ _ _ _ _ w529 _ _ _ _ _ _ _ _]
      tunnel: "Column Length" -> [_ _ _ _ _ w396 w431 _ _ _ _ _ _ _ _ _ _ w536 _ _ _ _ _ _ _ w718]
      frame "main", Default {
        w308 = 600.0 ("y")
        # "Advanced Settings"
        # "OSC Inputs"
        # "35"
        # "0"
        # "Output Cluster\n\n0 CO Conc %\n1 HC Conc %\n2 NOx Conc %\n3 O2 Conc %\n4 Propane/Propylene\n5 lambda P\n6 lambda I\n7 lambda D\n8 purge duration\n9 Target furnace lambda\n10 Log Interval\n11 Analysers\n12 Cycle Length\n13 Heat Load Control\n14 Ref Temp\n15 C Factor\n16 Target Heat Load\n17 Control TC 1\n18 Control TC 2"
        # "00 stop cmd\n01 Test Number\n02 Test Flow Rate\n03 Test Start Temperature\n04 Test Stop Temperature\n05 Furnace Ramp Rate\n06 Inlet Lambda\n07 Inlet O2\n08 Inlet Lambda Rich\n09 Inlet Lambda Lean\n10 Inlet Temperature\n11 NO SW"
        # "20"
        # "25"
        # "30"
        # "10"
        # "5"
        # "0"
        # "25"
        # "20"
        # "15"
        # "10"
        # "5"
        n118 = call-poly <vilib>:"Read From Spreadsheet File.vi"("file path (dialog if empty)"=w310) -> ("first row"=w309:dbl[])  [unwired: 6 in, 4 out]
        n119 = local read "output cluster"() -> (w329:T1)
        n120 = Multiply(x="Oxidation Duration (min)", y=w308) -> (x*y=w303:T2)
        n121 = Multiply(x="Oxidation Wait (min)", y=w308) -> (x*y=w302:T2)
        n122 = Multiply(x="Reduction Duration (min)", y=w308) -> (x*y=w301:T2)
        n123 = Multiply(x="Reduction Wait (min)", y=w308) -> (x*y=w300:T2)
        n124 = local read "Test number"() -> (w342:u16)
        n125 = Unbundle(w329) -> ("CO Concentration"=w322:dbl, "HC Concentration"=w321:dbl, "NOx Concentration"=w320:dbl, "O2 Concentration"=w319:dbl, "Propane"=w317:bool, "P"=w326:dbl, "I"=w325:dbl, "D"=w324:dbl, "Purge Duration"=w327:dbl, "Lambda Target"=w328:dbl, →"Log interval (seconds)":dbl, →"Analysers":u32, w313:dbl, "Heat Load Control"=w315:bool, w311:dbl[], "Text Alerts"=→"Text Alerts":bool, "Vehicle Name"=→"Vehicle Name":string, →"SMS Recipients":u32, "Directory"=→"Directory":string)
        "Cycle Length" <- w313
        "Heat Load Control" <- w315
        n126 = local read "HC Theory (%)"() -> (w318:T7)
        n127 = Boolean To (0,1)(Boolean=w317) -> (0, 1=w316:i16)
        n128 = Boolean To (0,1)(Boolean=w315) -> (0, 1=w312:i16)
        n129 = local read "Test Flow Rate(g/s)"() -> (w337:T2)
        n130 = local read "NO ppm Loff"() -> (w330:T2)
        n131 = local read "CO Theory (%)"() -> (w331:T7)
        n132 = local read "Inlet O2 (%)"() -> (w332:T2)
        n133 = Build Array (concatenate)("Stop Cmd", w342, w337, "Test Start Temperature (°C)", "Test Stop temperature (°C)", "Furnace Ramp Rate (°C/min)", w332, w331, w318, "Inlet LAMBDA Lean", "Inlet Temperature (°C)", "NO ppm SW", w330, "Nitrogen Injection (l/min)", w303, w302, w301, w300, w322, w321, w320, w319, w316, w326, w325, w324, w327, w328, w313, w312, w311, w309) -> (w334:T2[])
        n134 = shared-variable "RT CompactRIO Target\\Library 1.lvlib\\Control Variables"(w334) -> ()  [unwired: 1 in, 1 out]
        "Test number" <- "Select Test Type"
      }
      frame "start test" {
        w343 = FALSE
        n135 = property on="Pass" class="Bool (strict)"("Value"=w343) -> ()  [unwired: 2 in, 2 out]
        n136 = property on="Fail" class="Bool (strict)"("Value"=w343) -> ()  [unwired: 2 in, 2 out]
        n137 = local write "Pass"(w343) -> ()
        n138 = local write "Fail"(w343) -> ()
        n139 = shared-variable "RT CompactRIO Target\\Library 1.lvlib\\Enum 1"("Enum 1") -> ()  [unwired: 1 in, 1 out]
      }
      frame "clear table 1" {
        n140 = property on="Sub-Cycle Name" class="Str (strict)"("Value"="" ("Subcycle name")) -> ()  [unwired: 2 in, 2 out]
        n141 = local write "Ageing - Cycle Pattern"(string[][] [["", "0", "", "", "", "", "", "", "", "", "", "", ""], ["", "", "", "", "", "", "", "", "", "", "", "", ""], ["", "", "", "", "", "", "", "", "", "", "", "", ""], ["", "", "", "", "", "", "", "", "", "", "", "", ""], ["", "", "", "", "", "", "", "", "", "", "", "", ""], ["", "", "", "", "", "", "", "", "", "", "", "", ""], ["", "", "", "", "", "", "", "", "", "", "", "", ""], ["", "", "", "", "", "", "", "", "", "", "", "", ""], ["", "", "", "", "", "", "", "", "", "", "", "", ""], ["", "", "", "", "", "", "", "", "", "", "", "", ""], ["", "", "", "", "", "", "", "", "", "", "", "", ""], ["", "", "", "", "", "", "", "", "", "", "", "", ""], ["", "", "", "", "", "", "", "", "", "", "", "", ""], ["", "", "", "", "", "", "", "", "", "", "", "", ""], ["", "", "", "", "", "", "", "", "", "", "", "", ""], ["", "", "", "", "", "", "", "", "", "", "", "", ""], ["", "", "", "", "", "", "", "", "", "", "", "", ""], ["", "", "", "", "", "", "", "", "", "", "", "", ""], ["", "", "", "", "", "", "", "", "", "", "", "", ""], ["", "", "", "", "", "", "", "", "", "", "", "", ""], ["", "", "", "", "", "", "", "", "", "", "", "", ""], ["", "", "", "", "", "", "", "", "", "", "", "", ""], ["", "", "", "", "", "", "", "", "", "", "", "", ""], ["", "", "", "", "", "", "", "", "", "", "", "", ""], ["", "", "", "", "", "", "", "", "", "", "", "", ""], ["", "", "", "", "", "", "", "", "", "", "", "", ""], ["", "", "", "", "", "", "", "", "", "", "", "", ""], ["", "", "", "", "", "", "", "", "", "", "", "", ""], ["", "", "", "", "", "", "", "", "", "", "", "", ""], ["", "", "", "", "", "", "", "", "", "", "", "", ""], ["", "", "", "", "", "", "", "", "", "", "", "", ""]]) -> ()
        n142 = local write "Flag1"(FALSE) -> ()
      }
      frame "update list 1" {
        n143 = String To Path(string=w351) -> (path=w350:path)
        n144 = List Folder(path=w350, pattern="*.eyes") -> (filenames=w349:string[])  [unwired: 2 in, 3 out]
        n145 = property on="Cycle List" class="LstBox (strict)"("Item Names"=w349) -> ()  [unwired: 2 in, 2 out]
      }
      frame "save subc" {
        w355 = ".eyes" ("string")
        n146 = local read "Cycle Name"() -> (w354:T3)
        n147 = String To Path(string=w362) -> (path=w367:path)
        n148 = Equal?(x=w354, y="") -> (x = y?=w359:bool)
        n149 = List Folder(path=w367, pattern="*.eyes" ("string")) -> (filenames=w366:string[])  [unwired: 2 in, 3 out]
        n150 = Concatenate Strings(w354, w355) -> (w353:string)
        n151 = Concatenate Strings(w362, w354, w355) -> (w368:string)
        n152 = Search 1D Array(1D array=w366, element=w353) -> (index of element=w365:i32)  [unwired: 1 in]
        n153 = case shown="True" w359 {
          tunnel: [TRUE FALSE] -> w358
          frame False {
          }
          frame True {
            n154 = One Button Dialog(message="Insert file name!") -> ()  [unwired: 1 in, 1 out]
          }
        }
        n155 = String To Path(string=w368) -> (path=w361:path)
        n156 = Equal?(x=w365, y=-1) -> (x = y?=w363:bool)
        n157 = case shown="False" w363 {
          selector: w363 -> [_ w374]
          tunnel: [w372 w374] -> w357
          frame False {
            n158 = Two Button Dialog(message="A file with this name already exists!\nDo you want to overwrite?") -> (T button?=w372:bool)  [unwired: 2 in]
          }
          frame True {
          }
        }
        n159 = And(x=w357, y=w358) -> (x .and. y?=w356:bool)
        n160 = case shown="True" w356 {
          tunnel: w361 -> [_ w379]
          frame False {
          }
          frame True {
            n161 = local read "Ageing - Cycle Pattern"() -> (w378:string[][])
            n162 = call "Table check.vi"("Input table"=w378) -> ("Incomplete?"=w376:bool, "Length"=w377:i32)  [unwired: 9 in]
            n163 = case shown="False" w376 {
              tunnel: w378 -> [w387 _]
              tunnel: w379 -> [w386 _]
              tunnel: w377 -> [w385 _]
              tunnel: string[] [] -> [w384 _]
              frame False {
                n164 = for {
                  N: w385 -> [_]
                  tunnel: w387 -> [w394]
                  shift-right: [w391] -> w383
                  shift-left: w384 -> [w392]
                  i -> [w393]
                  n165 = Index Array(array=w394, index (row)=w393) -> (element=w390:string[])  [unwired: 1 in]
                  n166 = Delete From Array(array=w390, index=0) -> (array with subset deleted=w389:string[])  [unwired: 1 in, 1 out]
                  n167 = Build Array (concatenate)(w392, w389) -> (w391:string[])
                }
                n168 = Build Array (concatenate)("SubCycle Data File for EYECAT - do not modify", w383) -> (w381:string[])
                n169 = call-poly <vilib>:"Write To Spreadsheet File.vi"("1D data"=w381, "file path (dialog if empty)"=w386) -> ()  [unwired: 6 in, 1 out]
              }
              frame True {
                n170 = One Button Dialog(message="The table is incomplete!\nplease review and save again!") -> ()  [unwired: 1 in, 1 out]
              }
            }
            n171 = local write "Flag1"(FALSE) -> ()
          }
        }
      }
      frame "load subc" {
        n172 = local read "Flag1"() -> (w400:bool)
        n173 = case shown="True" w400 {
          tunnel: [w427 w429] -> w398
          tunnel: w399 -> [w427 w429]
          tunnel: [TRUE w428] -> w397
          frame False {
          }
          frame True {
            n174 = Two Button Dialog(message="The table has been modified.\nDo you want to continue?") -> (T button?=w428:bool)  [unwired: 2 in]
          }
        }
        n175 = case shown="True" w397 {
          tunnel: w398 -> [_ w401]
          tunnel: w396 -> [_ w402]
          frame False {
          }
          frame True {
            n176 = property on="Cycle List" class="LstBox (strict)"() -> ("Item Names"=w416:string[])  [unwired: 2 in, 2 out]
            n177 = Index Array(array=w416, index="Cycle List") -> (element=w405:string)
            n178 = Concatenate Strings(w401, w405) -> (w414:string)
            n179 = Search/Split String(string=w405, search string/char (-)=".") -> (substring before match=w403:string)  [unwired: 1 in, 2 out]
            n180 = String To Path(string=w414) -> (path=w413:path)
            n181 = local write "Cycle Name"(w403) -> ()
            n182 = call-poly <vilib>:"Read From Spreadsheet File.vi"("file path (dialog if empty)"=w413) -> ("first row"=w410:string[])  [unwired: 6 in, 4 out]
            n183 = Delete From Array(array=w410, length=1, index=0) -> (array with subset deleted=w407:string[])  [unwired: 1 out]
            n184 = Array Size(array=w407) -> (size(s)=w412:i32)
            n185 = Divide(x=w412, y=w402) -> (x/y=w406:dbl)
            n186 = for {
              N: w406 -> [_]
              shift-right: [w423] -> _
              shift-left: w407 -> [w425]
              tunnel: [w422] -> w411 mode=indexing
              tunnel: w402 -> [w417]
              i -> [w421]
              n187 = Increment(x=w421) -> (x+1=w420:i32)
              n188 = Delete From Array(array=w425, length=w417, index=0) -> (deleted portion=w418:string[], array with subset deleted=w423:string[])
              n189 = Number To Decimal String(number=w420) -> (decimal integer string=w419:string)  [unwired: 1 in]
              n190 = Build Array (concatenate)(w419, w418) -> (w422:string[])
            }
            n191 = local write "Ageing - Cycle Pattern"(w411) -> ()
          }
        }
      }
      frame "Export Cycle" {
        n192 = flat-sequence {
          tunnel: w432 -> [w435]
          tunnel: w431 -> [w433]
          frame #0 {
            n193 = case shown="True" TRUE {
              tunnel: w435 -> [_ w445]
              tunnel: w433 -> [_ w436]
              frame False {
              }
              frame True {
                n194 = property on="Cycle List" class="LstBox (strict)"() -> ("Item Names"=w437:string[])  [unwired: 2 in, 2 out]
                n195 = local read "Cycle List"() -> (w439:i32)
                n196 = Index Array(array=w437, index=w439) -> (element=w444:string)
                n197 = Concatenate Strings(w445, w444) -> (w453:string)
                n198 = Search/Split String(string=w444, search string/char (-)=".") -> (substring before match=w440:string)  [unwired: 1 in, 2 out]
                n199 = String To Path(string=w453) -> (path=w452:path)
                n200 = local write "Cycle Name"(w440) -> ()
                n201 = call-poly <vilib>:"Read From Spreadsheet File.vi"("file path (dialog if empty)"=w452) -> ("first row"=w450:string[])  [unwired: 6 in, 4 out]
                n202 = Delete From Array(array=w450, length=1, index=0) -> (array with subset deleted=w447:string[])  [unwired: 1 out]
                n203 = Array Size(array=w447) -> (size(s)=w451:i32)
                n204 = Divide(x=w451, y=w436) -> (x/y=w446:dbl)
                n205 = Concatenate Strings("c:\\Setup Files\\Exported\\", w440) -> (w442:string)
                n206 = String To Path(string=w442) -> (path=w438:path)
                n207 = for {
                  N: w446 -> [_]
                  shift-right: [w458] -> _
                  shift-left: w447 -> [w460]
                  tunnel: [w456] -> _ mode=indexing
                  tunnel: w438 -> [w457]
                  tunnel: w436 -> [w454]
                  n208 = Delete From Array(array=w460, length=w454, index=0) -> (deleted portion=w456:string[], array with subset deleted=w458:string[])
                  n209 = call-poly <vilib>:"Write To Spreadsheet File.vi"("append to file? (new file:F)"=TRUE, "1D data"=w456, "file path (dialog if empty)"=w457) -> ()  [unwired: 5 in, 1 out]
                }
              }
            }
          }
          frame #1 {
          }
        }
      }
      frame "delete subc" {
        n210 = Two Button Dialog(message="This operation will permanently delete this file!\nDo you want to continue?") -> (T button?=w462:bool)  [unwired: 2 in]
        n211 = case shown="True" w462 {
          tunnel: w463 -> [_ w468]
          frame False {
          }
          frame True {
            n212 = local read "Cycle List"() -> (w465:i32)
            n213 = property on="Cycle List" class="LstBox (strict)"() -> ("Item Names"=w466:string[])  [unwired: 2 in, 2 out]
            n214 = Index Array(array=w466, index=w465) -> (element=w470:string)
            n215 = Concatenate Strings(w468, w470) -> (w469:string)
            n216 = local write "Flag1"(FALSE) -> ()
            n217 = String To Path(string=w469) -> (path=w467:path)
            n218 = Delete(path (use dialog)=w467) -> ()  [unwired: 4 in, 3 out]
          }
        }
      }
      frame "clear table 2" {
      }
      frame "update list 2" {
      }
      frame "save cycle" {
      }
      frame "load cycle" {
      }
      frame "delete cycle" {
      }
      frame "calc HC CO" {
        n219 = local read "Sub-Cycle Pattern"() -> (w487:string[][])
        n220 = Index Array(array=w487, index (col) #1=3 ("disabled index (col)"), index (col) #2=4 ("index (col)"), index (col) #3=11 ("index (col)")) -> (element #1=w477:string[], element #2=w484:string[], element #3=w471:string[])  [unwired: 3 in]
        n221 = Array Size(array=w477) -> (size(s)=w475:i32)
        n222 = Search 1D Array(1D array=w477, element="") -> (index of element=w474:i32)  [unwired: 1 in]
        n223 = Equal?(x=w474, y=-1) -> (x = y?=w476:bool)
        n224 = Select(t=w475, s=w476, f=w474) -> (s? t:f=w473:i32)
        n225 = for {
          N: w473 -> [_]
          tunnel: [w498] -> w481 mode=indexing
          tunnel: [w497] -> w480 mode=indexing
          tunnel: w477 -> [w496] mode=indexing
          tunnel: w484 -> [w495] mode=indexing
          tunnel: w471 -> [w494] mode=indexing
          w493 = ""
          n226 = Not Equal?(x=w496, y=w493) -> (x != y?=w492:bool)
          n227 = Not Equal?(x=w495, y=w493) -> (x != y?=w491:bool)
          n228 = Not Equal?(x=w494, y=w493) -> (x != y?=w490:bool)
          n229 = Compound Arithmetic op=AND(w492, w491, w490) -> (w489:bool)
          n230 = case shown="True" w489 {
            tunnel: w496 -> [_ w527]
            tunnel: w495 -> [_ w526]
            tunnel: [w499 w523] -> w497
            tunnel: [w499 w522] -> w498
            tunnel: w494 -> [_ w500]
            frame False {
              w499 = ""
            }
            frame True {
              # "O2Eq"
              n231 = Fract/Exp String To Number(string=w500) -> (number=w501:dbl)  [unwired: 3 in, 1 out]
              n232 = Fract/Exp String To Number(string=w527) -> (number=w508:dbl)  [unwired: 3 in, 1 out]
              n233 = Fract/Exp String To Number(string=w526) -> (number=w504:dbl)  [unwired: 3 in, 1 out]
              n234 = Decrement(x=w508) -> (x-1=w509:dbl)
              n235 = Divide(x=w501, y=20000.0) -> (x/y=w502:dbl)
              n236 = Multiply(x=4.76, y=w508) -> (x*y=w513:dbl)
              n237 = Multiply(x=w509, y=100.0) -> (x*y=w511:dbl)
              n238 = Add(x=w504, y=w502) -> (x+y=w505:dbl)
              n239 = Add(x=0.33, y=w513) -> (x+y=w515:dbl)
              n240 = Divide(x=w511, y=w515) -> (x/y=w516:dbl)
              n241 = Subtract(x=w505, y=w516) -> (x-y=w518:dbl)
              n242 = Multiply(x=w518, y=2.0) -> (x*y=w506:dbl)
              n243 = Divide(x=w518, y=5.0) -> (x/y=w507:dbl)
              n244 = Number To Fractional String(number=w507, width (-)=i16 6, precision (6)=i16 3) -> (F-format string=w522:string)  [unwired: 1 in]
              n245 = Number To Fractional String(number=w506, width (-)=i16 6, precision (6)=i16 2) -> (F-format string=w523:string)  [unwired: 1 in]
            }
          }
        }
        n246 = Replace Array Subset(array=w487, new element #1=w481, index (col) #1=5 ("disabled index (col)"), new element #2=w480, index (col) #2=6 ("disabled index (col)")) -> (w485:string[][])  [unwired: 2 in]
        n247 = local write "Sub-Cycle Pattern"(w485) -> ()
      }
      frame "Total time calc" {
      }
      frame "update Cycle pattern " {
      }
      frame "load cycle name" {
      }
      frame "load test array" {
        n248 = call-poly <vilib>:"Read From Spreadsheet File.vi"("file path (dialog if empty)"=w529) -> ("first row"=w533:dbl[])  [unwired: 6 in, 4 out]
        n249 = local read "Cycle Name"() -> (w538:T3)
        n250 = Index Array(array=w533, index=15) -> (element=w532:dbl)
        n251 = Number To Boolean Array(number=w532) -> (Boolean array=w530:bool[])
        n252 = Equal?(x=w538, y="") -> (x = y?=w535:bool)
        n253 = Index Array(array=w530, index=2) -> (element=w528:bool)
        n254 = case shown="True" w535 {
          selector: w535 -> [w540 _]
          tunnel: [FALSE TRUE] -> w537
          tunnel: w536 -> [_ w545]
          tunnel: w528 -> [_ w544]
          frame False {
            n255 = case shown="False" w540 {
              frame False {
                n256 = One Button Dialog(message="Incomplete Data!\nReview the cycle pattern!") -> ()  [unwired: 1 in, 1 out]
              }
              frame True {
              }
            }
          }
          frame True {
            n257 = case shown="True" w544 {
              tunnel: [w561 w622] -> w547
              tunnel: [w560 w621] -> w546
              tunnel: w545 -> [w558 w627]
              tunnel: [dbl[] [] w623] -> w543
              frame False {
                # "Pre-Cat V\nBypass V\nEvac-1"
                # "CO\nAir-1\nAir-2\nHC-1\nHC-2\nNO\nAir-Bal\nHC-Bal\nO2"
                n258 = local read "Cycle Name"() -> (w562:T3)
                n259 = Concatenate Strings("C:\\Setup Files\\Ageing Cycles\\Omega\\", w562, ".eyes" ("string")) -> (w579:string)
                n260 = String To Path(string=w579) -> (path=w580:path)
                n261 = call-poly <vilib>:"Read From Spreadsheet File.vi"("file path (dialog if empty)"=w580) -> ("all rows"=w563:dbl[][])  [unwired: 6 in, 4 out]
                n262 = Transpose 2D Array(2D array=w563) -> (transposed array=w569:dbl[][])
                n263 = Array Size(array=w569) -> (size(s)=w568:i32[])
                n264 = Index Array(array=w568) -> (element=w576:i32)  [unwired: 1 in]
                n265 = Reshape Array(w563, w576) -> (w567:dbl[])
                n266 = Decrement(x=w576) -> (x-1=w577:i32)
                n267 = Delete From Array(array=w567, length=1, index=0) -> (array with subset deleted=w565:dbl[])  [unwired: 1 out]
                n268 = Divide(x=w577, y=w558) -> (x/y=w559:dbl)
                n269 = for {
                  N: w559 -> [_]
                  shift-right: [w598] -> _
                  shift-left: w565 -> [w600]
                  tunnel: [w597] -> w575 mode=indexing
                  tunnel: [w596] -> w574 mode=indexing
                  tunnel: [w595] -> w573 mode=indexing
                  tunnel: [w594] -> w572 mode=indexing
                  tunnel: [w593] -> w571 mode=indexing
                  tunnel: [w592] -> w570 mode=indexing
                  tunnel: [w591] -> w553 mode=indexing
                  tunnel: [w589] -> w554 mode=indexing
                  tunnel: [w587] -> w555 mode=indexing
                  tunnel: [w586] -> w556 mode=indexing
                  tunnel: [w585] -> w557 mode=indexing
                  tunnel: [w588] -> w552 mode=indexing
                  tunnel: w558 -> [w584]
                  tunnel: [w583] -> w550 mode=indexing
                  tunnel: [w582] -> w549 mode=indexing
                  n270 = Delete From Array(array=w600, length=w584, index=0) -> (deleted portion=w590:dbl[], array with subset deleted=w598:dbl[])
                  n271 = Index Array(array=w590) -> (element #1=w597:dbl, element #2=w596:dbl, element #3=w595:dbl, element #4=w594:dbl, element #5=w593:dbl, element #6=w592:dbl, element #7=w591:dbl, element #8=w589:dbl, element #9=w588:dbl, element #10=w587:dbl, element #11=w586:dbl, element #12=w585:dbl, element #13=w583:dbl, element #14=w582:dbl)  [unwired: 14 in]
                }
                n272 = Build Array (concatenate)(w559, w553, w554, w555, w556, w557, w550, w549) -> (w560:dbl[])
                "Valve Array" <- w560
                n273 = Build Array (concatenate)(w559, w575, w574, w573, w572, w571, w570, w552) -> (w561:dbl[])
                "MFC Array" <- w561
              }
              frame True {
                n274 = local read "Cycle Name"() -> (w626:T3)
                n275 = Concatenate Strings("C:\\Setup Files\\Ageing Cycles\\Omicron\\", w626, ".eyes" ("string")) -> (w629:string)
                n276 = String To Path(string=w629) -> (path=w628:path)
                n277 = call-poly <vilib>:"Read From Spreadsheet File.vi"("file path (dialog if empty)"=w628) -> ("all rows"=w638:dbl[][])  [unwired: 6 in, 4 out]
                n278 = Transpose 2D Array(2D array=w638) -> (transposed array=w632:dbl[][])
                n279 = Array Size(array=w632) -> (size(s)=w633:i32[])
                n280 = Index Array(array=w633) -> (element=w631:i32)  [unwired: 1 in]
                n281 = Reshape Array(w638, w631) -> (w634:dbl[])
                n282 = Decrement(x=w631) -> (x-1=w630:i32)
                n283 = Delete From Array(array=w634, length=1, index=0) -> (array with subset deleted=w636:dbl[])  [unwired: 1 out]
                n284 = Divide(x=w630, y=w627) -> (x/y=w620:dbl)
                n285 = for {
                  N: w620 -> [_]
                  shift-right: [w660] -> _
                  shift-left: w636 -> [w662]
                  tunnel: [w659] -> w619 mode=indexing
                  tunnel: [w658] -> w618 mode=indexing
                  tunnel: [w657] -> w617 mode=indexing
                  tunnel: [w656] -> w616 mode=indexing
                  tunnel: [w655] -> w615 mode=indexing
                  tunnel: [w654] -> w614 mode=indexing
                  tunnel: [w653] -> w613 mode=indexing
                  tunnel: [w651] -> w612 mode=indexing
                  tunnel: [w649] -> w610 mode=indexing
                  tunnel: [w648] -> w609 mode=indexing
                  tunnel: [w647] -> w608 mode=indexing
                  tunnel: [w650] -> w611 mode=indexing
                  tunnel: w627 -> [w646]
                  tunnel: [w645] -> w607 mode=indexing
                  tunnel: [w644] -> w606 mode=indexing
                  tunnel: [w643] -> w605 mode=indexing
                  tunnel: [w642] -> w604 mode=indexing
                  tunnel: [w641] -> w603 mode=indexing
                  tunnel: [w640] -> w602 mode=indexing
                  tunnel: [w639] -> w601 mode=indexing
                  n286 = Delete From Array(array=w662, length=w646, index=0) -> (deleted portion=w652:dbl[], array with subset deleted=w660:dbl[])
                  n287 = Index Array(array=w652) -> (element #1=w659:dbl, element #2=w658:dbl, element #3=w657:dbl, element #4=w656:dbl, element #5=w655:dbl, element #6=w654:dbl, element #7=w653:dbl, element #8=w651:dbl, element #9=w650:dbl, element #10=w649:dbl, element #11=w648:dbl, element #12=w647:dbl, element #13=w645:dbl, element #14=w644:dbl, element #15=w643:dbl, element #16=w642:dbl, element #17=w641:dbl, element #18=w640:dbl, element #19=w639:dbl)  [unwired: 19 in]
                }
                n288 = Build Array (concatenate)(w620, w619, w618, w617, w616, w615, w614) -> (w622:dbl[])
                n289 = Build Array (concatenate)(w620, w613, w612, w611, w610, w609, w608) -> (w623:dbl[])
                n290 = Build Array (concatenate)(w620, w607, w606, w605, w604, w603, w602, w601) -> (w621:dbl[])
              }
            }
            n291 = shared-variable "RT CompactRIO Target\\Library 1.lvlib\\Inject_Arrays_System"(w546) -> ()  [unwired: 1 in, 1 out]
            n292 = shared-variable "RT CompactRIO Target\\Library 1.lvlib\\Inject_Arrays_Cat-2"(w543) -> ()  [unwired: 1 in, 1 out]
            n293 = shared-variable "RT CompactRIO Target\\Library 1.lvlib\\Inject_Arrays_Cat-1"(w547) -> ()  [unwired: 1 in, 1 out]
          }
        }
        "Test Compiled" <- w537
      }
      frame "convert to num" {
        n294 = local read "EditPos Subc"() -> (w666:T4)
        n295 = Unbundle By Name(w666) -> ("Row"=w667:i32, "Column"=w664:i32)
        n296 = Equal?(x=w664, y=7) -> (x = y?=w663:bool)
        n297 = case shown="False" w663 {
          tunnel: w667 -> [_ w672]
          tunnel: w664 -> [_ w670]
          tunnel: w666 -> [_ _]
          frame True {
          }
          frame False {
            n298 = local read "Sub-Cycle Pattern"() -> (w669:string[][])
            n299 = call "Conv to num.vi"("Column"=w670, "Row"=w672, "Array"=w669) -> ("result string"=w671:string)  [unwired: 8 in]
            n300 = Replace Array Subset(array=w669, new element=w671, index (row)=w672, index (col)=w670) -> (w668:string[][])
            n301 = local write "Sub-Cycle Pattern"(w668) -> ()
          }
        }
      }
      frame "check scycle name" {
        n302 = local read "Cycle Name"() -> (w673:T3)
        n303 = call <vilib>:"Search and Replace Pattern.vi"("string"=w673, "regular expression (\"\")"="[^0-9a-zA-Z ]" ("format string"), "replace string (\"\")"="", "replace all? (F)"=TRUE) -> ("result string"=w679:string)  [unwired: 1 in, 1 out]
        n304 = Not Equal?(x=w679, y=w673) -> (x != y?=w678:bool)
        n305 = case shown="False" w678 {
          tunnel: w679 -> [w680 w681]
          tunnel: [w680 w681] -> w674
          frame False {
          }
          frame True {
            n306 = One Button Dialog(message="Unsuitable character for the file name!") -> ()  [unwired: 1 in, 1 out]
          }
        }
        n307 = local write "Cycle Name"(w674) -> ()
      }
      frame "check cycle name" {
        n308 = local read "Cycle Name"() -> (w683:T3)
        n309 = call <vilib>:"Search and Replace Pattern.vi"("string"=w683, "regular expression (\"\")"="[^0-9a-zA-Z ]" ("format string"), "replace string (\"\")"="", "replace all? (F)"=TRUE) -> ("result string"=w689:string)  [unwired: 1 in, 1 out]
        n310 = Not Equal?(x=w689, y=w683) -> (x != y?=w688:bool)
        n311 = case shown="False" w688 {
          tunnel: w689 -> [w690 w691]
          tunnel: [w690 w691] -> w684
          frame False {
          }
          frame True {
            n312 = One Button Dialog(message="Unsuitable character for the file name!") -> ()  [unwired: 1 in, 1 out]
          }
        }
        n313 = local write "Cycle Name"(w684) -> ()
      }
      frame "Multigas connect" {
        # "add here logic to verify the user requirements and the machine state\n0 - not connected\n1 - MKS1 & Ext An Up\n2 - MKS2 & Ext An Dn\n3 - MKS 1 & 2  & Ext An Up & Dn"
        n314 = flat-sequence {
          frame #0 {
            "Connected?" <- TRUE
          }
        }
      }
      frame "Multigas disconnect" {
      }
      frame "Leak Test" {
        n315 = call "Press_Test.vi"() -> ("Reset Button"=w694:bool)  [unwired: 11 in]
        n316 = local write "Leak Test"(w694) -> ()
      }
      frame "Import Cycle" {
        n317 = call-poly <vilib>:"Read From Spreadsheet File.vi"("delimiter (\\t)"="," ("delimiter (\\t)")) -> ("all rows"=w699:string[][])  [unwired: 6 in, 4 out]
        n318 = Array Size(array=w699) -> (size(s)=w701:i32[])
        n319 = Index Array(array=w701, index #1=0 ("index")) -> (element #1=w698:i32, element #2=w697:i32)  [unwired: 1 in]
        n320 = for {
          N: w698 -> [_]
          shift-right: [w711] -> _
          shift-left: w699 -> [w713]
          tunnel: [w704] -> w695 mode=indexing
          tunnel: w697 -> [w706]
          i -> [w710]
          n321 = Delete From Array(array=w713, length=1, index (row)=0 ("index")) -> (deleted portion=w707:string[][], array with subset deleted=w711:string[][])  [unwired: 1 in]
          n322 = Increment(x=w710) -> (x+1=w709:i32)
          n323 = Reshape Array(w707, w706) -> (w705:string[])
          n324 = Number To Decimal String(number=w709) -> (decimal integer string=w703:string)  [unwired: 1 in]
          n325 = Build Array (concatenate)(w703, w705) -> (w704:string[])
        }
        n326 = local write "Ageing - Cycle Pattern"(w695) -> ()
        n327 = local write "Cycle Name"(T3 "" ("Drive Cycle Name")) -> ()
      }
      frame "Display Graph" {
        n328 = local read "Cycle Name"() -> (w728:T3)
        n329 = local read "Graph Cycle Box"() -> (w717:string)
        n330 = local read "Graph Cycle Box 2"() -> (w715:string)
        n331 = Octal String To Number(4:w717) -> (0:w716:u32)  [unwired: 2 in, 1 out]
        n332 = Concatenate Strings(w729, w728, ".eyes" ("string")) -> (w737:string)
        n333 = String To Path(string=w737) -> (path=w736:path)
        n334 = call-poly <vilib>:"Read From Spreadsheet File.vi"("file path (dialog if empty)"=w736) -> ("all rows"=w738:dbl[][])  [unwired: 6 in, 4 out]
        n335 = Octal String To Number(4:w715) -> (0:w714:u32)  [unwired: 2 in, 1 out]
        n336 = Transpose 2D Array(2D array=w738) -> (transposed array=w731:dbl[][])
        n337 = Array Size(array=w731) -> (size(s)=w732:i32[])
        n338 = Index Array(array=w732) -> (element=w730:i32)  [unwired: 1 in]
        n339 = Reshape Array(w738, w730) -> (w733:dbl[])
        n340 = Decrement(x=w730) -> (x-1=w724:i32)
        n341 = Delete From Array(array=w733, length=1, index=0) -> (array with subset deleted=w723:dbl[])  [unwired: 1 out]
        n342 = Divide(x=w724, y=w718) -> (x/y=w725:dbl)
        n343 = for {
          N: w725 -> [_]
          shift-right: [w749] -> _
          shift-left: w723 -> [w743]
          tunnel: [w748] -> w726 mode=indexing
          tunnel: [w746] -> _ mode=indexing
          tunnel: w716 -> [w745]
          tunnel: [w744] -> w719 mode=indexing
          tunnel: w714 -> [w741]
          tunnel: w718 -> [w740]
          i -> [w747]
          n344 = Increment(x=w747) -> (x+1=w746:i32)
          n345 = Delete From Array(array=w743, length=w740, index=0) -> (deleted portion=w742:dbl[], array with subset deleted=w749:dbl[])
          n346 = Index Array(array=w742, index=w745) -> (element=w748:dbl)
          n347 = Index Array(array=w742, index=w741) -> (element=w744:dbl)
        }
        n348 = call "Convert to Dynamic Data"("Array"=w726) -> ("Dynamic Data Type"=w727:dynamicdata)  [unwired: 3 in]
        n349 = call "Convert to Dynamic Data2"("Array"=w719) -> ("Dynamic Data Type"=w721:dynamicdata)  [unwired: 3 in]
        n350 = Merge Signals(w727) -> (→"MFC Graph 5":dynamicdata)
        n351 = Merge Signals(w721) -> (→"MFC Graph 6":dynamicdata)
      }
    }
    n352 = local read "stop 2"() -> (w293:bool)
  }
  n353 = node-c288(nitl_modes."Discard missed periods, maintain original phase" ("Mode")) -> (w77:T12)  [unwired: 4 in]
  n354 = node-c288(w50) -> (w71:T12)  [unwired: 3 in]
  n355 = node-c288(i64 100 ("Period")) -> (w23:T12)  [unwired: 3 in]
  n356 = timed-loop {
    timing: w77 -> [_]
    timing-out: [_] -> w76
    shift-right: [w933] -> _
    shift-left: path "" -> [w930]
    shift-right: [w950] -> _
    shift-left: w47 -> [w973]
    shift-right: [w924] -> _
    shift-left: _ -> [w955]
    shift-right: [w943] -> _
    shift-left: w47 -> [w753]
    shift-right: [w944] -> _
    shift-left: w47 -> [w945]
    tunnel: w61 -> [w850]
    shift-right: [w766] -> _
    shift-left: w47 -> [w765]
    shift-right: [w762] -> _
    shift-left: 0 ("Counter Out") -> [w761]
    shift-right: [w756] -> _
    shift-left: FALSE -> [w755]
    stop <- w972 stop-if-true
    w793 = 17 ("length")
    (unwired) i32[] [0, 8, 13, 18, 3, 9, 14, 5, 10, 15, 21, 20, 6, 11, 16, 23, 1, 7, 12, 22] ("appended array")
    # "True OMEGA False Maxcat"
    n357 = node-c288() -> (→"Finished Late? [i-1]":bool, →"Iteration Duration":i64)  [unwired: 1 in, 1 out]
    n358 = shared-variable "RT CompactRIO Target\\Library 1.lvlib\\DATA"() -> (w971:dbl[])  [unwired: 1 in, 1 out]
    n359 = call-poly <vilib>:"Read From Spreadsheet File.vi"("file path (dialog if empty)"=w850) -> ("first row"=w758:dbl[])  [unwired: 6 in, 4 out]
    n360 = Type Cast(type=w971, x=w971) -> (*(type *) &x=w978:dbl[])
    n361 = Delete From Array(array=w978, length=4, index=0) -> (deleted portion=w975:dbl[], array with subset deleted=w785:dbl[])
    n362 = Index Array(array=w975) -> (element #1=w924:dbl, element #2=w958:dbl, element #3=w759:dbl, element #4=w954:dbl)  [unwired: 4 in]
    "Error" <- w759
    "Loop Number" <- w924
    n363 = local read "ETAS Out"() -> (w783:dbl[])
    n364 = To Unsigned Long Integer(number=w954) -> (unsigned 32bit integer=w953:u32)
    n365 = Index Array(array=w758, index=15) -> (element=w797:dbl)
    n366 = Number To Boolean Array(number=w953) -> (Boolean array=w966:bool[])
    n367 = Number To Boolean Array(number=w797) -> (Boolean array=w796:bool[])
    n368 = Index Array(array=w966) -> (element #2=w964:bool, element #3=w963:bool, element #4=w952:bool, element #5=→"ExtAnUp":bool, element #6=→"ExtAnDn":bool)  [unwired: 6 in, 1 out]
    "Extractor Fan On" <- w952
    n369 = Build Array (concatenate)(w785, w783) -> (w784:dbl[])
    n370 = Index Array(array=w796, index=2) -> (element=w756:bool)
    n371 = local read "File Directory"() -> (w851:string)
    n372 = Or(x=w964, y=w963) -> (x .or. y?=→"Doors Open":bool)
    n373 = Not(x=w952) -> (.not. x?=→"Doors Unlocked":bool)
    n374 = case shown="0, Default" w958 {
      tunnel: [w1019 TRUE FALSE] -> w957
      tunnel: [w1020 FALSE TRUE] -> w956
      frame 0, Default {
        n375 = local read "Pass"() -> (w1020:bool)
        n376 = local read "Fail"() -> (w1019:bool)
      }
      frame 1 {
      }
      frame 2 {
      }
    }
    "Pass" <- w956
    "Fail" <- w957
    n377 = Equal?(x=w924, y=4.0) -> (x = y?=w923:bool)
    n378 = Equal?(x=w924, y=5.0) -> (x = y?=w922:bool)
    n379 = case shown="0, Default" w924 {
      tunnel: [w1000 w1003 w1006 w1009 TRUE FALSE] -> w853
      tunnel: [w1000 w1003 w1006 TRUE w1012 w1017] -> w854
      tunnel: [TRUE w1003 w1006 w1009 w1012 w1017] -> w856
      tunnel: [w1000 TRUE TRUE w1009 w1012 w1017] -> w855
      tunnel: [w1000 w1003 w1006 w1009 w1012 TRUE] -> w852
      tunnel: w765 -> [w999 w1002 _ w1008 w1011 w1015]
      tunnel: [w999 w1002 0.0 ("y") w1008 w1011 w1015] -> w764
      frame 0, Default {
        w1000 = FALSE
      }
      frame 1 {
        w1003 = FALSE
      }
      frame 2 {
        w1006 = FALSE
      }
      frame 3 {
        w1009 = FALSE
      }
      frame 4 {
        w1012 = FALSE
        n380 = local write "Stop Cmd"(T2 0.0 ("Stop Cmd")) -> ()
      }
      frame 5 {
        w1017 = FALSE
      }
    }
    "Cool Down" <- w853
    "Test In Progress" <- w854
    "Standby" <- w856
    "Warm Up" <- w855
    "STBY" <- w856
    "WMUP" <- w855
    "TEST" <- w854
    "COOL" <- w853
    "OFF" <- w852
    n381 = case shown="False" w756 {
      tunnel: ["Time\tFlow Vent g/s\tFlow Vane g/s\tETAS 1\tETAS 2\tUEGO 1\tUEGO 2\tTank P\tTC1\tTC2\tTC3\tTC4\tTC5\tTC6\tTC Mopup\tTC Tank\tTC Vent\tTC Vane\tTC Bearing 1\tTC Bearing 2\tTC HExA\tTC HExB\tTC HExC\tTC HExD\tTC Furn\tP Time\tTime Step\tCat HL Control\tHeat Load 1\tAgeing Time\tRemaining Time\tRemaining Time Sec\t% Complete\tHeat Load 2\tAgeing Time\tRemaining Time\tRemaining Time Sec\t% Complete\tTime Remaining\tPT1\tPT2\tPT3\tPT4\tCumulative Electricity Consumption\tETAS 1\tETAS 2\tETAS O2 1\tETAS O2 2\tCO\tCO2\tCO L\tO2\tSO2\tTHC\tNOx\tCO2\tCO\tO2\tTHC\t\tNOx\tCO2\tCO\tO2\tTHC\tNOx\tCO 500\tCO\tH2O\tC3H6\tC3H8\tCO2\tNO\tNOx\tNO2\tNH3\r\n" ("Heading string 2") "Time\tFlow Vent g/s\tFlow Vane g/s\tETAS 1\tETAS 2\tUEGO 1\tUEGO 2\tTank P\tTC1\tTC2\tTC3\tTC4\tTC5\tTC6\tTC Mopup\tTC Tank\tTC Vent\tTC Vane\tTC Bearing 1\tTC Bearing 2\tTC HExA\tTC HExB\tTC HExC\tTC HExD\tTC Furn\tP Time\tTime Step\tCat HL Control\tHeat Load 1\tAgeing Time\tRemaining Time\tRemaining Time Sec\t% Complete\tHeat Load 2\tAgeing Time\tRemaining Time\tRemaining Time Sec\t% Complete\tTime Remaining\tPT1\tPT2\tPT3\tPT4\tCumulative Electricity Consumption\tETAS 1\tETAS 2\tETAS O2 1\tETAS O2 2\tCO\tCO2\tCO L\tO2\tSO2\tTHC\tNOx\tCO2\tCO\tO2\tTHC\t\tNOx\tCO2\tCO\tO2\tTHC\tNOx\tCO 500\tCO\tH2O\tC3H6\tC3H8\tCO2\tNO\tNOx\tNO2\tNH3\r\n" ("Heading string 2")] -> w792
      frame False {
      }
      frame True {
      }
    }
    n382 = Or(x=w923, y=w922) -> (x .or. y?=w925:bool)
    n383 = Array Subset(array=w784, index=26 ("length"), length=11 ("index")) -> (w861:dbl[])
    n384 = String To Path(string=w851) -> (path=w951:path)
    n385 = case shown="False" w925 {
      frame False {
      }
      frame True {
        n386 = local write "Enum 1"(i16 0 ("Enum 1")) -> ()
        n387 = local write "Start Test"(FALSE ("Start Test")) -> ()
      }
    }
    n388 = local read "Cycle Length"() -> (w858:dbl)
    n389 = Not Equal?(x=w951, y=w930) -> (x != y?=w980:bool)
    n390 = local read "Heat Load Control"() -> (w857:bool)
    n391 = Select(t=w951, s=w980, f=w930) -> (s? t:f=w981:path)
    n392 = local write "Stop Test"(w853) -> ()
    n393 = property on="OFF" class="Bool (strict)"("Visible"=w852) -> ()  [unwired: 2 in, 2 out]
    n394 = case shown="True" FALSE {
      tunnel: w981 -> [w1062 w1066]
      tunnel: [w1062 w1065] -> w979
      tunnel: w792 -> [_ w1063]
      frame False {
      }
      frame True {
        # "setting up the header"
        n395 = Build Array(w1063) -> (w1064:string[])
        n396 = call-poly <vilib>:"Write To Spreadsheet File.vi"("1D data"=w1064, "file path (dialog if empty)"=w1066) -> ("new file path (Not A Path if cancelled)"=w1065:path)  [unwired: 6 in]
      }
    }
    n397 = call "Test_Complete.vi"("Cycle Length"=w858, "array"=w861, "Heatload"=w857) -> ("% Complete"=→"% Complete":u8, "Time Remaining"=→"Time Remaining":dbl)  [unwired: 7 in]
    n398 = Less?(x=w924, y=w955) -> (x < y?=w776:bool)
    n399 = Not Equal?(x=w755, y=w756) -> (x != y?=w757:bool)
    n400 = Equal To 0?(x=w759) -> (x = 0?=w935:bool)
    n401 = Equal To 0?(x=w924) -> (x = 0?=w934:bool)
    n402 = Build Array(w935, w934) -> (w961:bool[])
    n403 = local write "Stopped?"(w776) -> ()
    n404 = property on="COOL" class="Bool (strict)"("Visible"=w853) -> ()  [unwired: 2 in, 2 out]
    n405 = Boolean Array To Number(Boolean array=w961) -> (number=w960:u32)
    n406 = property on="WMUP" class="Bool (strict)"("Visible"=w855) -> ()  [unwired: 2 in, 2 out]
    n407 = property on="STBY" class="Bool (strict)"("Visible"=w856) -> ()  [unwired: 2 in, 2 out]
    n408 = property on="TEST" class="Bool (strict)"("Visible"=w854) -> ()  [unwired: 2 in, 2 out]
    n409 = Index Array(array=i32[] [24, 0, 25, 23, 22, 19, 20, 26, 27, 28, 29, 11, 12, 14, 23, 13, 15, 16, 17, 18, 19, 20, 21, 22] ("appended array")) -> (element #1=w831:i32, element #2=w821:i32, element #3=w820:i32, element #4=w819:i32, element #5=w817:i32, element #6=w816:i32, element #7=w815:i32, element #8=w814:i32, element #9=w813:i32, element #10=w804:i32, element #11=w803:i32)  [unwired: 11 in]
    n410 = case shown="0, Default" w960 {
      tunnel: [w1053 w1054 w1059 w1061] -> _
      tunnel: [w1053 w1054 w1059 w1061] -> _
      tunnel: [w1053 w1054 w1059 w1061] -> _
      tunnel: [w1053 w1054 w1057 w1061] -> w959
      tunnel: [T14."Enabled" ("Disabled") T14."Enabled" ("Disabled") w1057 w1061] -> _
      tunnel: [FALSE FALSE FALSE TRUE] -> w949
      frame 0, Default {
        w1053 = T14."Disabled and Grayed Out" ("Disabled")
      }
      frame 1 {
        w1054 = T14."Disabled and Grayed Out" ("Disabled")
      }
      frame 2 {
        w1057 = T14."Enabled" ("Disabled")
        w1059 = T14."Disabled and Grayed Out" ("Disabled")
      }
      frame 3 {
        w1061 = T14."Enabled" ("Disabled")
        (unwired) T14."Disabled and Grayed Out" ("Disabled")
      }
    }
    n411 = case shown="True" w757 {
      tunnel: w756 -> [_ w989]
      frame False {
      }
      frame True {
        n412 = property on="Omicron" class="Bool (strict)"("Val(Sgnl)"=w989) -> ()  [unwired: 2 in, 2 out]
      }
    }
    n413 = Index Array(array=w758, index #1=w831, index #2=w821, index #3=w820, index #4=w819, index #5=w817, index #6=w816, index #7=w815, index #8=w814, index #9=w813, index #10=w804, index #11=w803) -> (element #1=w829:dbl, element #3=w826:dbl, element #4=w823:dbl, element #5=w818:dbl, element #6=w812:dbl, element #7=w810:dbl, element #8=w808:dbl, element #9=w806:dbl, element #10=w802:dbl, element #11=w800:dbl)  [unwired: 1 out]
    n414 = Decrement(x=w800) -> (x-1=w799:dbl)
    n415 = Decrement(x=w802) -> (x-1=w801:dbl)
    n416 = Equal?(x=w924, y=2.0) -> (x = y?=w942:bool)
    n417 = Equal?(x=w924, y=3.0) -> (x = y?=w939:bool)
    n418 = local read "Mexa 1"() -> (w788:dbl[])
    n419 = local read "Mexa 2"() -> (w789:dbl[])
    n420 = local read "Mexa 3"() -> (w790:dbl[])
    n421 = Equal?(x=w924, y=4.0) -> (x = y?=w751:bool)
    n422 = local read "MKS 1"() -> (w791:dbl[])
    n423 = Index Array(array=i32[] [0, 1, 6, 2, 3, 4, 5, 54, 55, 9, 10, 11, 12, 14, 23, 13, 15, 16, 17, 18, 19, 20, 21, 22] ("appended array")) -> (element #1=w919:i32, element #2=w918:i32, element #3=w913:i32, element #4=w912:i32, element #5=w911:i32, element #6=w910:i32, element #7=w907:i32)  [unwired: 7 in]
    n424 = Decrement(x=w806) -> (x-1=w805:dbl)
    n425 = Decrement(x=w808) -> (x-1=w807:dbl)
    n426 = Compound Arithmetic op=OR(w942, w939, w751) -> (w941:bool)
    n427 = Decrement(x=w810) -> (x-1=w809:dbl)
    n428 = property on="Purge System" class="Bool"("DisabledEnum"=w959) -> ()  [unwired: 2 in, 2 out]
    n429 = property class="VI"("Front Panel.Closeable"=w949) -> ()  [unwired: 2 in, 2 out]
    n430 = Decrement(x=w812) -> (x-1=w811:dbl)
    n431 = case shown="True" w751 {
      tunnel: w753 -> [w986 w987]
      tunnel: [w986 w988] -> w752
      frame False {
      }
      frame True {
        n432 = Increment(x=w987) -> (x+1=w988:T2)
      }
    }
    n433 = Decrement(x=w818) -> (x-1=w822:dbl)
    n434 = Decrement(x=w823) -> (x-1=w824:dbl)
    n435 = Build Array (concatenate)(w788, w789, w790, w791) -> (w787:dbl[])
    n436 = Decrement(x=w826) -> (x-1=w825:dbl)
    n437 = Decrement(x=w829) -> (x-1=w827:dbl)
    n438 = Decrement(x=w793) -> (x-1=w828:i32)
    n439 = Delete From Array(array=w784, length=w793, index=7) -> (deleted portion=w843:dbl[], array with subset deleted=w781:dbl[])
    n440 = local read "% Complete"() -> (w771:u8)
    n441 = local read "Cool Down"() -> (w767:bool)
    n442 = local read "Log Test Data"() -> (w936:bool)
    n443 = Build Array (concatenate)(w784, w787) -> (w864:dbl[])
    n444 = Equal To 0?(x=w764) -> (x = 0?=w768:bool)
    n445 = Index Array(array=w784, index #1=w919, index #2=w918, index #3=w913, index #4=w912, index #5=w911, index #6=w910, index #7=w907) -> (element #1=w929:dbl, element #2=w928:dbl, element #3=w782:dbl, element #4=w915:dbl, element #5=w914:dbl, element #6=w909:dbl, element #7=w786:dbl)
    "Pressure" <- w782
    "Flow 1" <- w929
    "Flow 2" <- w928
    n446 = Index Array(array=w781, index #1=26 ("index"), index #2=27 ("index")) -> (element #1=w778:dbl, element #2=w777:dbl)
    n447 = Index Array(array=w843, index #7=w827, index #8=w828, index #9=w825, index #10=w824, index #11=w822, index #12=w811, index #13=w809, index #14=w807, index #15=w805, index #16=w801, index #17=w799) -> (element #1=w849:dbl, element #2=w848:dbl, element #3=w847:dbl, element #4=w846:dbl, element #5=w845:dbl, element #6=w844:dbl, element #7=w842:dbl, element #8=w841:dbl, element #9=w840:dbl, element #10=w839:dbl, element #11=w838:dbl, element #12=w837:dbl, element #13=w836:dbl, element #14=w835:dbl, element #15=w834:dbl, element #16=w833:dbl, element #17=w832:dbl)  [unwired: 6 in]
    "TC 1" <- w849
    "TC 3" <- w847
    "TC 4" <- w846
    "TC 5" <- w845
    "TC 6" <- w844
    "TC 2" <- w848
    n448 = Greater Or Equal?(x=w771, y=u8 100) -> (x >= y?=w769:bool)
    n449 = for {
      tunnel: w864 -> [w1068] mode=indexing
      tunnel: [w1067] -> w982 mode=indexing
      n450 = Number To Fractional String(number=w1068, precision (6)=i16 3) -> (F-format string=w1067:string)  [unwired: 2 in]
    }
    n451 = Compound Arithmetic op=AND(w769, w767, w768) -> (w763:bool)
    n452 = And(x=w936, y=w941) -> (x .and. y?=w985:bool)
    "Log?" <- w985
    n453 = Not Equal To 0?(x=w759) -> (x != 0?=w760:bool)
    n454 = Not Equal?(x=w759, y=w973) -> (x != y?=w974:bool)
    n455 = local read "Text Alerts"() -> (w772:bool)
    "SMS" <- w772
    n456 = local read "SMS Recipients"() -> (w774:u32)
    n457 = local read "Vehicle Name"() -> (w775:string)
    n458 = Index Array(array=i32[] [0, 8, 14, 19, 3, 9, 15, 5, 10, 16, 21, 20, 6, 11, 17, 23, 1, 7, 13, 22] ("appended array")) -> (element #1=w889:i32, element #2=w883:i32, element #3=w882:i32, element #4=w881:i32, element #5=w880:i32, element #6=w879:i32, element #7=w878:i32, element #8=w877:i32, element #9=w876:i32, element #10=w875:i32, element #11=w874:i32, element #12=w873:i32, element #13=w872:i32, element #14=w871:i32, element #15=w870:i32, element #16=w869:i32, element #17=w868:i32, element #18=w867:i32, element #19=w866:i32, element #20=w865:i32)  [unwired: 20 in]
    n459 = local read "File Name"() -> (w773:T3)
    n460 = Index Array(array=w787, index #1=w889, index #2=w883, index #3=w882, index #4=w881, index #5=w880, index #6=w879, index #7=w878, index #8=w877, index #9=w876, index #10=w875, index #11=w874, index #12=w873, index #13=w872, index #14=w871, index #15=w870, index #16=w869, index #17=w868, index #18=w867, index #19=w866, index #20=w865) -> (element #1=w905:dbl, element #2=w904:dbl, element #3=w903:dbl, element #4=w902:dbl, element #5=w901:dbl, element #6=w900:dbl, element #7=w899:dbl, element #8=w898:dbl, element #9=w897:dbl, element #10=w896:dbl, element #11=w895:dbl, element #12=w894:dbl, element #13=w893:dbl, element #14=w892:dbl, element #15=w891:dbl, element #16=w890:dbl, element #17=w887:dbl, element #18=w886:dbl, element #19=w885:dbl, element #20=w884:dbl)
    n461 = case shown="True" w985 {
      tunnel: w979 -> [w1072 w1080]
      tunnel: [w1072 w1092] -> w933
      tunnel: w982 -> [_ w1088]
      tunnel: w752 -> [_ w1081]
      tunnel: w945 -> [w1071 w1076]
      tunnel: [w1071 w1078] -> w944
      tunnel: [w1070 w1077] -> w943
      frame False {
        n462 = local read "Log interval (seconds)"() -> (w1070:T2)
      }
      frame True {
        n463 = Get Date/Time In Seconds() -> (seconds since 1Jan1904=w1089:timestamp)
        n464 = Decrement(x=w1081) -> (x-1=w1082:T2)
        n465 = Less Than 0?(x=w1082) -> (x < 0?=w1083:bool)
        n466 = Equal To 0?(x=w1082) -> (x = 0?=w1084:bool)
        n467 = Build Array(w1083, w1084) -> (w1085:bool[])
        n468 = Path To String(path=w1080) -> (string=w1075:string)
        "File name" <- w1075
        n469 = Format Date/Time String(time format string (%c)="%d/%m/%y %H:%M:%S", seconds (now)=w1089) -> (date/time string=w1090:string)  [unwired: 1 in]
        n470 = Boolean Array To Number(Boolean array=w1085) -> (number=w1086:u32)
        n471 = case shown="0, Default" w1086 {
          tunnel: w1081 -> [w1099 w1100 _]
          tunnel: [w1098 w1100 w1103] -> w1077
          tunnel: w1075 -> [w1097 w1102 w1106]
          tunnel: [w1094 w1102 w1104] -> w1079
          tunnel: [w1093 w1101 w1105] -> w1078
          tunnel: w1076 -> [w1093 w1101 w1109]
          frame 0, Default {
            n472 = Number To Decimal String(number=w1093) -> (decimal integer string=w1095:string)  [unwired: 1 in]
            n473 = call <vilib>:"Space Constant.vi"() -> ("String"=w1096:string)
            n474 = Decrement(x=w1099) -> (x-1=w1098:T2)
            n475 = Concatenate Strings(w1097, w1096, w1095) -> (w1094:string)
          }
          frame 1 {
          }
          frame 2 {
            n476 = Increment(x=w1109) -> (x+1=w1105:dbl)
            n477 = local read "Log interval (seconds)"() -> (w1103:T2)
            n478 = Number To Decimal String(number=w1105) -> (decimal integer string=w1107:string)  [unwired: 1 in]
            n479 = call <vilib>:"Space Constant.vi"() -> ("String"=w1108:string)
            n480 = Concatenate Strings(w1106, w1108, w1107) -> (w1104:string)
          }
        }
        n481 = Build Array (concatenate)(w1090, w1088) -> (w1074:string[])
        n482 = String To Path(string=w1079) -> (path=w1073:path)
        n483 = call-poly <vilib>:"Write To Spreadsheet File.vi"("append to file? (new file:F)"=TRUE, "1D data"=w1074, "file path (dialog if empty)"=w1073) -> ("new file path (Not A Path if cancelled)"=w1092:path)  [unwired: 5 in]
      }
    }
    n484 = case shown="True" w760 {
      tunnel: w759 -> [w1027 w1039]
      tunnel: w974 -> [w1030 w1035]
      tunnel: [w1026 w1039] -> w950
      tunnel: w772 -> [_ w1038]
      tunnel: w774 -> [_ w1037]
      tunnel: w775 -> [_ w1036]
      tunnel: [0 ("Counter Out") w1043] -> w762
      tunnel: w761 -> [_ w1040]
      frame False {
        n485 = Equal To 0?(x=w1027) -> (x = 0?=w1031:bool)
        n486 = And(x=w1031, y=w1030) -> (x .and. y?=w1029:bool)
        n487 = case shown="True" w1029 {
          frame False {
          }
          frame True {
            w1034 = FALSE ("Ack hard alarm!")
            n488 = property on="System Alarm" class="Bool (strict)"("Value"=w1034) -> ()  [unwired: 2 in, 2 out]
            n489 = property on="Hard Alarm" class="Bool (strict)"("Value"=w1034) -> ()  [unwired: 2 in, 2 out]
            n490 = property on="System Alarm" class="Bool (strict)"("Value"=w1034) -> ()  [unwired: 2 in, 2 out]
          }
        }
        n491 = case shown="True" "Acknowledge" {
          tunnel: [w1032 0.0 ("Numeric")] -> w1026
          tunnel: w1027 -> [w1032 _]
          frame False {
          }
          frame True {
          }
        }
      }
      frame True {
        n492 = local read "Table"() -> (w1041:string[][])
        n493 = call "Error list.vi"("New Alarm?"=w1035, "Vehicle"=w1036, "Error array in"=w1041, "SMS Recipients"=w1037, "Send SMS"=w1038, "Error code"=w1039, "Counter In"=w1040) -> ("Hard alarm?"=w1044:bool, "Counter Out"=w1043:i32, "Error array out"=w1042:string[][])  [unwired: 2 in]
        "Hard Alarm" <- w1044
        n494 = Not(x=w1044) -> (.not. x?=w1046:bool)
        "Soft Alarm" <- w1046
        n495 = Or(x=w1046, y=w1044) -> (x .or. y?=→"System Alarm":bool)
        n496 = case shown="False" w1046 {
          frame False {
          }
          frame True {
            n497 = property on="Alarm ack" class="Bool"("DisabledEnum"=T14."Enabled" ("Disabled")) -> ()  [unwired: 2 in, 2 out]
          }
        }
        n498 = case shown="True" w1035 {
          tunnel: w1042 -> [_ w1049]
          frame False {
          }
          frame True {
            n499 = local write "Table"(w1049) -> ()
            n500 = property on="Tab Control" class="TabCtl (strict)"("Value"=6) -> ()  [unwired: 2 in, 2 out]
          }
        }
        n501 = local write "Acknowledge"(FALSE ("Acknowledge")) -> ()
      }
    }
    n502 = case shown="True" w763 {
      tunnel: w775 -> [_ w992]
      tunnel: w774 -> [_ w993]
      tunnel: w773 -> [_ w994]
      tunnel: w772 -> [_ _]
      tunnel: [w990 1.0 ("y")] -> w766
      tunnel: w764 -> [w990 _]
      frame False {
      }
      frame True {
        n503 = call "Test Complete Core.vi"("Vehicle"=w992, "SMS Recipients"=w993, "File Name"=w994) -> ()  [unwired: 9 in]
      }
    }
    n504 = Merge Signals(w929, w928) -> (→"Flow Rate (g/s)":dynamicdata)
    n505 = Merge Signals(w782) -> (→"System Pressure (kPa)":dynamicdata)
    n506 = Merge Signals(w915, w914, w909, w786, w778, w777) -> (→"Lambda":dynamicdata)
    n507 = Merge Signals(w905, w904, w903, w902) -> (→"CO Concentration (%)":dynamicdata)
    n508 = Merge Signals(w901, w900, w899) -> (→"O2 Concentration (%)":dynamicdata)
    n509 = Merge Signals(w898, w897, w896, w895, w894) -> (→"HC Concentration (ppm)":dynamicdata)
    n510 = Merge Signals(w893, w892, w891, w890) -> (→"NO Concentration (ppm)":dynamicdata)
    n511 = Merge Signals(w887, w886, w885, w884) -> (→"CO2 Concentration (%)":dynamicdata)
    n512 = Merge Signals(w849, w848, w847, w846, w845, w844) -> (→"Sample Temperatures (°C)":dynamicdata)
    n513 = Merge Signals(w842, w841, w840) -> (→"System Temperatures (°C)":dynamicdata)
    n514 = Merge Signals(w839, w838, w837, w836) -> (→"Gas Flow Measurement Temperatures (°C)":dynamicdata)
    n515 = Merge Signals(w835, w834, w833, w832) -> (→"Heat Exchanger Temperatures (°C)":dynamicdata)
    n516 = local read "stop 2"() -> (w972:bool)
    n517 = node-c288() -> ()  [unwired: 1 in, 1 out]
  }
  n518 = timed-loop {
    timing: w71 -> [_]
    timing-out: [_] -> w70
    shift-right: [w1115] -> _
    shift-left: path "" -> [w1154]
    shift-right: [w1118] -> _
    shift-left: w44 -> [w1114]
    shift-right: [w1117] -> _
    shift-left: w44 -> [w1116]
    stop <- _ stop-if-true
    n519 = node-c288() -> ()  [unwired: 1 in, 1 out]
    n520 = shared-variable "RT CompactRIO Target\\Library 1.lvlib\\DATA_2"() -> (w1128:dbl[])  [unwired: 1 in, 1 out]
    n521 = local read "Directory"() -> (w1123:string)
    n522 = Path To String(path=path "C:/DATA LOG" ("File Path")) -> (string=w1126:string)
    n523 = Equal?(x=w1123, y="") -> (x = y?=w1124:bool)
    n524 = case shown="True" w1124 {
      tunnel: w1126 -> [_ w1221]
      tunnel: [w1220 w1221] -> w1125
      tunnel: w1123 -> [w1220 _]
      frame False {
      }
      frame True {
      }
    }
    n525 = case shown="\"CO\", Default" "Graph 1 Box" {
      tunnel: [0 ("index") 1 ("index") 2 ("index") 3 ("index") 4 ("index") 5 ("index") 6 ("index") 7 ("index") 8 ("index") 9 ("index") 10 ("index")] -> w1166
      tunnel: [11 ("index") 12 ("index") 13 ("index") 14 ("index") 15 ("index") 16 ("index") 17 ("index") 18 ("index") 19 ("index") 20 ("index") 21 ("index")] -> w1173
      frame "CO", Default {
      }
      frame "HC Cycle 1" {
      }
      frame "Air Cycle 1" {
      }
      frame "NO" {
      }
      frame "N2" {
      }
      frame "Air Bal" {
      }
      frame "HC Bal" {
      }
      frame "Air Cycle 2" {
      }
      frame "N2-2" {
      }
      frame "HC Cycle 2" {
      }
      frame "O2" {
      }
    }
    n526 = case shown="\"CO\", Default" "Graph 2 Box" {
      tunnel: [11 ("index") 12 ("index") 13 ("index") 14 ("index") 15 ("index") 16 ("index") 17 ("index") 18 ("index") 19 ("index") 20 ("index") 21 ("index")] -> w1143
      tunnel: [0 ("index") 1 ("index") 2 ("index") 3 ("index") 4 ("index") 5 ("index") 6 ("index") 7 ("index") 8 ("index") 9 ("index") 10 ("index")] -> w1142
      frame "CO", Default {
      }
      frame "HC Cycle 1" {
      }
      frame "Air Cycle 1" {
      }
      frame "NO" {
      }
      frame "N2" {
      }
      frame "Air Bal" {
      }
      frame "HC Bal" {
      }
      frame "Air Cycle 2" {
      }
      frame "N2-2" {
      }
      frame "HC Cycle 2" {
      }
      frame "O2" {
      }
    }
    n527 = case shown="\"CO\", Default" "Graph 3 Box" {
      tunnel: [11 ("index") 12 ("index") 13 ("index") 14 ("index") 15 ("index") 16 ("index") 17 ("index") 18 ("index") 19 ("index") 20 ("index") 21 ("index")] -> w1136
      tunnel: [0 ("index") 1 ("index") 2 ("index") 3 ("index") 4 ("index") 5 ("index") 6 ("index") 7 ("index") 8 ("index") 9 ("index") 10 ("index")] -> w1137
      frame "CO", Default {
      }
      frame "HC Cycle 1" {
      }
      frame "Air Cycle 1" {
      }
      frame "NO" {
      }
      frame "N2" {
      }
      frame "Air Bal" {
      }
      frame "HC Bal" {
      }
      frame "Air Cycle 2" {
      }
      frame "N2-2" {
      }
      frame "HC Cycle 2" {
      }
      frame "O2" {
      }
    }
    n528 = case shown="\"CO\", Default" "Graph 4 Box" {
      tunnel: [11 ("index") 12 ("index") 13 ("index") 14 ("index") 15 ("index") 16 ("index") 17 ("index") 18 ("index") 19 ("index") 20 ("index") 21 ("index")] -> w1134
      tunnel: [0 ("index") 1 ("index") 2 ("index") 3 ("index") 4 ("index") 5 ("index") 6 ("index") 7 ("index") 8 ("index") 9 ("index") 10 ("index")] -> w1135
      frame "CO", Default {
      }
      frame "HC Cycle 1" {
      }
      frame "Air Cycle 1" {
      }
      frame "NO" {
      }
      frame "N2" {
      }
      frame "Air Bal" {
      }
      frame "HC Bal" {
      }
      frame "Air Cycle 2" {
      }
      frame "N2-2" {
      }
      frame "HC Cycle 2" {
      }
      frame "O2" {
      }
    }
    n529 = case shown="\"CO\", Default" "Graph 5 Box" {
      tunnel: [11 ("index") 12 ("index") 13 ("index") 14 ("index") 15 ("index") 16 ("index") 17 ("index") 18 ("index") 19 ("index") 20 ("index") 21 ("index")] -> w1132
      tunnel: [0 ("index") 1 ("index") 2 ("index") 3 ("index") 4 ("index") 5 ("index") 6 ("index") 7 ("index") 8 ("index") 9 ("index") 10 ("index")] -> w1133
      frame "CO", Default {
      }
      frame "HC Cycle 1" {
      }
      frame "Air Cycle 1" {
      }
      frame "NO" {
      }
      frame "N2" {
      }
      frame "Air Bal" {
      }
      frame "HC Bal" {
      }
      frame "Air Cycle 2" {
      }
      frame "N2-2" {
      }
      frame "HC Cycle 2" {
      }
      frame "O2" {
      }
    }
    n530 = case shown="\"CO\", Default" "Graph 6 Box" {
      tunnel: [11 ("index") 12 ("index") 13 ("index") 14 ("index") 15 ("index") 16 ("index") 17 ("index") 18 ("index") 19 ("index") 20 ("index") 21 ("index")] -> w1130
      tunnel: [0 ("index") 1 ("index") 2 ("index") 3 ("index") 4 ("index") 5 ("index") 6 ("index") 7 ("index") 8 ("index") 9 ("index") 10 ("index")] -> w1131
      frame "CO", Default {
      }
      frame "HC Cycle 1" {
      }
      frame "Air Cycle 1" {
      }
      frame "NO" {
      }
      frame "N2" {
      }
      frame "Air Bal" {
      }
      frame "HC Bal" {
      }
      frame "Air Cycle 2" {
      }
      frame "N2-2" {
      }
      frame "HC Cycle 2" {
      }
      frame "O2" {
      }
    }
    n531 = Index Array(array=w1128, index #1=w1166, index #2=w1173) -> (element #1=w1168:dbl, element #2=w1167:dbl)
    n532 = Index Array(array=w1128, index #1=w1142, index #2=w1143) -> (element #1=w1165:dbl, element #2=w1164:dbl)
    n533 = Index Array(array=w1128, index #1=w1137, index #2=w1136) -> (element #1=w1163:dbl, element #2=w1162:dbl)
    n534 = Index Array(array=w1128, index #1=w1135, index #2=w1134) -> (element #1=w1161:dbl, element #2=w1160:dbl)
    n535 = Index Array(array=w1128, index #1=w1133, index #2=w1132) -> (element #1=w1152:dbl, element #2=w1153:dbl)
    n536 = Index Array(array=w1128, index #1=w1131, index #2=w1130) -> (element #1=w1151:dbl, element #2=w1150:dbl)
    n537 = for {
      tunnel: w1128 -> [w1360] mode=indexing
      tunnel: [w1359] -> w1121 mode=indexing
      n538 = Number To Fractional String(number=w1360, precision (6)=i16 3) -> (F-format string=w1359:string)  [unwired: 2 in]
    }
    n539 = Concatenate Strings(w1125, "\\" ("string"), "File Name") -> (w1146:string)
    "File Directory" <- w1146
    n540 = Merge Signals(w1168, w1167) -> (→"MFC Graph 1":dynamicdata)
    n541 = Merge Signals(w1165, w1164) -> (→"MFC Graph 2":dynamicdata)
    n542 = Merge Signals(w1163, w1162) -> (→"MFC Graph 3":dynamicdata)
    n543 = Merge Signals(w1161, w1160) -> (→"MFC Graph 4":dynamicdata)
    n544 = Merge Signals(w1152, w1153) -> (→"MFC Graph 5":dynamicdata)
    n545 = Merge Signals(w1151, w1150) -> (→"MFC Graph 6":dynamicdata)
    n546 = Concatenate Strings(w1146, "_MFC" ("string")) -> (w1174:string)
    n547 = String To Path(string=w1174) -> (path=w1155:path)
    n548 = local read "ETAS Out"() -> (w1127:dbl[])
    n549 = Not Equal?(x=w1155, y=w1154) -> (x != y?=w1157:bool)
    n550 = shared-variable "RT CompactRIO Target\\Library 1.lvlib\\Analyser_Data"(w1127) -> ()  [unwired: 1 in, 1 out]
    n551 = Select(t=w1155, s=w1157, f=w1154) -> (s? t:f=w1156:path)
    n552 = case shown="True" w1157 {
      tunnel: w1156 -> [w1332 w1336]
      tunnel: [w1332 w1335] -> w1120
      tunnel: "Time\tCO Delivered\tHC Delivered\tAir Delivered\tNO Delivered\tN2 Delivered\tAir Bal Delivered\tHC Bal Delivered\tAir 2 Delivered\tN2 2 Delivered\tHC 2 Delivered\tO2 Delivered\r\n" ("Heading string 2") -> [_ w1333]
      frame False {
      }
      frame True {
        # "setting up the header"
        n553 = Build Array(w1333) -> (w1334:string[])
        n554 = call-poly <vilib>:"Write To Spreadsheet File.vi"("1D data"=w1334, "file path (dialog if empty)"=w1336) -> ("new file path (Not A Path if cancelled)"=w1335:path)  [unwired: 6 in]
      }
    }
    n555 = local read "Log?"() -> (w1119:bool)
    n556 = case shown="True" w1119 {
      tunnel: w1120 -> [w1180 w1189]
      tunnel: [w1180 w1200] -> w1115
      tunnel: w1121 -> [_ w1196]
      tunnel: w1114 -> [_ w1190]
      tunnel: w1116 -> [w1179 w1185]
      tunnel: [w1179 w1187] -> w1117
      tunnel: [w1177 w1186] -> w1118
      frame False {
        n557 = local read "Log interval (seconds)"() -> (w1178:T2)
        n558 = Multiply(x=w1178, y=T2 10.0) -> (x*y=w1177:T2)
      }
      frame True {
        n559 = Get Date/Time In Seconds() -> (seconds since 1Jan1904=w1197:timestamp)
        n560 = Decrement(x=w1190) -> (x-1=w1181:T2)
        n561 = Less Than 0?(x=w1181) -> (x < 0?=w1191:bool)
        n562 = Equal To 0?(x=w1181) -> (x = 0?=w1192:bool)
        n563 = Build Array(w1191, w1192) -> (w1193:bool[])
        n564 = Path To String(path=w1189) -> (string=w1184:string)
        n565 = Format Date/Time String(time format string (%c)="%d/%m/%y %H:%M:%S", seconds (now)=w1197) -> (date/time string=w1198:string)  [unwired: 1 in]
        n566 = Boolean Array To Number(Boolean array=w1193) -> (number=w1194:u32)
        n567 = case shown="2" w1194 {
          tunnel: w1181 -> [w1207 w1208 _]
          tunnel: [w1206 w1208 w1213] -> w1186
          tunnel: w1184 -> [w1205 w1210 w1216]
          tunnel: [w1202 w1210 w1214] -> w1188
          tunnel: [w1201 w1209 w1215] -> w1187
          tunnel: w1185 -> [w1201 w1209 w1219]
          frame 0, Default {
            n568 = Number To Decimal String(number=w1201) -> (decimal integer string=w1203:string)  [unwired: 1 in]
            n569 = call <vilib>:"Space Constant.vi"() -> ("String"=w1204:string)
            n570 = Decrement(x=w1207) -> (x-1=w1206:T2)
            n571 = Concatenate Strings(w1205, w1204, w1203) -> (w1202:string)
          }
          frame 1 {
          }
          frame 2 {
            n572 = Increment(x=w1219) -> (x+1=w1215:dbl)
            n573 = Number To Decimal String(number=w1215) -> (decimal integer string=w1217:string)  [unwired: 1 in]
            n574 = local read "Log interval (seconds)"() -> (w1211:T2)
            n575 = call <vilib>:"Space Constant.vi"() -> ("String"=w1218:string)
            n576 = Concatenate Strings(w1216, w1218, w1217) -> (w1214:string)
            n577 = Multiply(x=w1211, y=T2 10.0) -> (x*y=w1213:T2)
          }
        }
        n578 = Build Array (concatenate)(w1198, w1196) -> (w1183:string[])
        n579 = String To Path(string=w1188) -> (path=w1182:path)
        n580 = call-poly <vilib>:"Write To Spreadsheet File.vi"("append to file? (new file:F)"=TRUE, "1D data"=w1183, "file path (dialog if empty)"=w1182) -> ("new file path (Not A Path if cancelled)"=w1200:path)  [unwired: 5 in]
      }
    }
    n581 = node-c288() -> ()  [unwired: 1 in, 1 out]
  }
  n582 = timed-loop {
    timing: w23 -> [_]
    timing-out: [_] -> w22
    shift-right: [w1364] -> _
    shift-left: dbl[] [] ("Array of Double") -> [w1392]
    shift-right: [w1368] -> _
    shift-left: T3 "" ("File Name") -> [w1366]
    shift-right: [w1386] -> _
    shift-left: w18 -> [w1367]
    shift-right: [w1385] -> _
    shift-left: w18 -> [w1375]
    stop <- _ stop-if-true
    # "Data Logging For OSC Test"
    n583 = node-c288() -> ()  [unwired: 1 in, 1 out]
    n584 = local read "File Name"() -> (w1368:T3)
    n585 = flat-sequence {
      tunnel: w1392 -> [w1418]
      tunnel: w1367 -> [w1419]
      tunnel: w1375 -> [w1420]
      tunnel: w1368 -> [w1415]
      tunnel: path "C:/DATA LOG" ("File Path") -> [w1421]
      tunnel: [w1421] -> w1374
      tunnel: [w1416] -> w1373
      tunnel: [w1420] -> w1372
      tunnel: [w1419] -> w1371
      tunnel: [w1418] -> w1370
      tunnel: [w1414] -> w1369
      tunnel: w1366 -> [w1413]
      tunnel: [w1412] -> w1365
      tunnel: [w1430] -> w1383
      tunnel: [w1429] -> w1382
      tunnel: [w1428] -> w1381
      tunnel: [w1427] -> w1380
      tunnel: [w1426] -> w1379
      tunnel: [w1425] -> w1378
      tunnel: [w1423] -> w1377
      tunnel: [w1422] -> w1376
      tunnel: w1374 -> [w1430]
      tunnel: w1373 -> [w1429]
      tunnel: w1372 -> [w1428]
      tunnel: w1371 -> [w1427]
      tunnel: w1370 -> [w1426]
      tunnel: w1369 -> [w1425]
      tunnel: w1365 -> [w1422]
      tunnel: [w1431] -> w1399
      tunnel: [w1445] -> w1398
      tunnel: [w1444] -> w1397
      tunnel: [w1432] -> w1396
      tunnel: [w1435] -> w1395
      tunnel: [w1441] -> w1394
      tunnel: [w1439] -> w1391
      tunnel: [w1437] -> w1384
      tunnel: w1383 -> [w1445]
      tunnel: w1382 -> [w1444]
      tunnel: w1381 -> [w1442]
      tunnel: w1380 -> [w1440]
      tunnel: w1379 -> [w1439]
      tunnel: w1378 -> [w1438]
      tunnel: w1377 -> [w1433]
      tunnel: w1376 -> [w1432]
      tunnel: [w1453] -> w1408
      tunnel: [w1461] -> w1407
      tunnel: [w1463] -> w1406
      tunnel: [w1462] -> w1405
      tunnel: [w1460] -> w1402
      tunnel: [w1450] -> w1401
      tunnel: w1399 -> [w1453]
      tunnel: w1398 -> [w1463]
      tunnel: w1397 -> [w1462]
      tunnel: w1396 -> [w1460]
      tunnel: w1395 -> [w1458]
      tunnel: w1394 -> [w1457]
      tunnel: [w1456] -> w1393
      tunnel: w1391 -> [w1454]
      tunnel: [w1452] -> w1390
      tunnel: [w1451] -> w1387
      tunnel: w1384 -> [w1459]
      tunnel: [w1488] -> w1411
      tunnel: [w1483] -> w1410
      tunnel: w1408 -> [w1488]
      tunnel: w1407 -> [w1482]
      tunnel: w1406 -> [w1481]
      tunnel: w1405 -> [w1480]
      tunnel: [w1478] -> w1404
      tunnel: [w1477] -> w1403
      tunnel: w1402 -> [w1476]
      tunnel: w1401 -> [w1475]
      tunnel: [w1474] -> w1400
      tunnel: w1393 -> [w1473]
      tunnel: w1390 -> [w1472]
      tunnel: [w1472] -> w1389
      tunnel: [w1471] -> w1388
      tunnel: w1387 -> [w1471]
      tunnel: w1411 -> [w1489]
      tunnel: w1410 -> [w1496]
      tunnel: w1404 -> [w1493]
      tunnel: w1403 -> [w1492]
      tunnel: w1400 -> [w1495]
      tunnel: w1389 -> [w1491]
      tunnel: w1388 -> [w1490]
      tunnel: [w1491] -> w1386
      tunnel: [w1490] -> w1385
      tunnel: [w1489] -> w1364
      frame #0 {
        n586 = local read "Loop Number"() -> (w1412:dbl)
        n587 = Concatenate Strings(w1415, "_OSC" ("string")) -> (w1416:string)
        n588 = Equal?(x=w1415, y=w1413) -> (x = y?=w1414:bool)
      }
      frame #1 {
        n589 = Equal?(x=1.0, y=w1422) -> (x = y?=w1423:bool)
      }
      frame #2 {
        n590 = shared-variable "RT CompactRIO Target\\Library 1.lvlib\\OSC"() -> (w1431:dbl[])  [unwired: 1 in, 1 out]
        n591 = case shown="False" w1433 {
          tunnel: [w1448 u16 0 ("Test number")] -> w1435
          tunnel: w1442 -> [w1448 _]
          frame False {
          }
          frame True {
          }
        }
        n592 = case shown="False" w1438 {
          tunnel: [u16 0 ("Test number") w1447] -> w1441
          tunnel: w1440 -> [_ w1447]
          frame False {
          }
          frame True {
          }
        }
        n593 = Equal To 0?(x=w1435) -> (x = 0?=w1436:bool)
        n594 = Equal?(x=4.0, y=w1432) -> (x = y?=w1434:bool)
        n595 = And(x=w1436, y=w1434) -> (x .and. y?=w1437:bool)
      }
      frame #3 {
        n596 = case shown="True" w1459 {
          tunnel: w1457 -> [w1466 w1470]
          tunnel: [w1466 w1469] -> w1452
          tunnel: [w1465 w1468] -> w1461
          tunnel: w1458 -> [w1464 _]
          tunnel: [w1464 u16 1 ("Test number")] -> w1451
          frame False {
            n597 = Number To Decimal String(number=w1466) -> (decimal integer string=w1465:string)  [unwired: 1 in]
          }
          frame True {
            n598 = Increment(x=w1470) -> (x+1=w1469:u16)
            n599 = Number To Decimal String(number=w1469) -> (decimal integer string=w1468:string)  [unwired: 1 in]
          }
        }
        n600 = local read "Test number"() -> (w1450:u16)
        n601 = Not Equal?(x=w1454, y=w1453) -> (x != y?=w1455:bool[])
        n602 = Boolean Array To Number(Boolean array=w1455) -> (number=w1456:u64)
      }
      frame #4 {
        w1479 = 3.0 ("y")
        n603 = Path To String(path=w1481) -> (string=w1487:string)
        n604 = Not Equal To 0?(x=w1473) -> (x != 0?=w1474:bool)
        n605 = call <vilib>:"Space Constant.vi"() -> ("String"=w1484:string)
        n606 = Concatenate Strings(w1487, "\\" ("string"), w1480, w1484, w1482) -> (w1485:string)
        n607 = Equal?(x=w1476, y=w1479) -> (x = y?=w1478:bool)
        n608 = Equal?(x=w1479, y=w1475) -> (x = y?=w1477:bool)
        n609 = String To Path(string=w1485) -> (path=w1483:path)
      }
      frame #5 {
        n610 = Compound Arithmetic op=AND(w1495, w1493, w1492) -> (w1494:bool)
        n611 = case shown="True" w1494 {
          tunnel: w1489 -> [_ w1500]
          tunnel: w1496 -> [_ w1498]
          frame False {
          }
          frame True {
            w1501 = 13 ("length")
            n612 = for {
              tunnel: w1500 -> [w1515] mode=indexing
              tunnel: [w1514] -> w1504 mode=indexing
              n613 = Number To Fractional String(number=w1515, precision (6)=i16 3) -> (F-format string=w1514:string)  [unwired: 2 in]
            }
            n614 = Array Size(array=w1504) -> (size(s)=w1502:i32)
            n615 = Divide(x=w1502, y=w1501) -> (x/y=w1503:dbl)
            n616 = for {
              N: w1503 -> [_]
              shift-right: [w1511] -> _
              shift-left: w1504 -> [w1513]
              tunnel: [w1510] -> w1497 mode=indexing
              tunnel: w1501 -> [w1505]
              i -> [w1509]
              n617 = Increment(x=w1509) -> (x+1=w1508:i32)
              n618 = Delete From Array(array=w1513, length=w1505, index=0) -> (deleted portion=w1506:string[], array with subset deleted=w1511:string[])
              n619 = Number To Decimal String(number=w1508) -> (decimal integer string=w1507:string)  [unwired: 1 in]
              n620 = Build Array (concatenate)(w1507, w1506) -> (w1510:string[])
            }
            "OSC Results" <- w1497
            n621 = call-poly <vilib>:"Write To Spreadsheet File.vi"("append to file? (new file:F)"=FALSE, "2D data"=w1497, "file path (dialog if empty)"=w1498) -> ()  [unwired: 5 in, 1 out]
          }
        }
      }
    }
    n622 = node-c288() -> ()  [unwired: 1 in, 1 out]
  }
  n623 = while {
    tunnel: w93 -> [w1549]
    shift-right: [w1547] -> _
    shift-left: _ -> [w1546]
    shift-right: [w1544] -> _
    shift-left: T5."MAIN" ("Tab Control") -> [w1543]
    shift-right: [w1532] -> _
    shift-left: w68 -> [w1525]
    shift-right: [w1533] -> _
    shift-left: TRUE -> [w1526]
    shift-right: [w1531] -> _
    shift-left: w68 -> [w1520]
    shift-right: [w1530] -> _
    shift-left: w68 -> [w1521]
    shift-right: [w1529] -> _
    shift-left: w68 -> [w1522]
    shift-right: [w1528] -> _
    shift-left: w68 -> [w1523]
    shift-right: [w1527] -> _
    shift-left: w68 -> [w1524]
    tunnel: w13 -> [w1519]
    stop <- w1545 stop-if-true
    n624 = event shown="[28] \"Adv Settings\": Value Change" {
      selector: _ -> [_ _ _ _ _ _ _ _ _ _ _ _ _ _ _ _ _ _ _ _ _ _ _ _ _ _ _ _ _ _ _ _ _ _ _ _ _ _ _ _ _ _ _]
      dyn-events: _ -> [_ _ _ _ _ _ _ _ _ _ _ _ _ _ _ _ _ _ _ _ _ _ _ _ _ _ _ _ _ _ _ _ _ _ _ _ _ _ _ _ _ _ _]
      timeout: 100 -> [_ _ _ _ _ _ _ _ _ _ _ _ _ _ _ _ _ _ _ _ _ _ _ _ _ _ _ _ _ _ _ _ _ _ _ _ _ _ _ _ _ _ _]
      tunnel: w1549 -> [w1568 w1570 _ w1579 w1588 w1590 w1601 w1608 w1619 w1623 w1634 w1639 w1642 w1646 w1658 w1659 _ _ _ _ w1703 w1714 _ w1758 w1782 _ w1796 _ _ _ _ _ _ _ _ _ _ _ w1844 w1850 w1851 _ _]
      tunnel: [w1566 w1569 _ w1580 w1587 _ w1600 w1607 w1618 w1621 w1629 w1636 w1641 w1645 _ _ _ _ _ _ _ _ _ _ _ _ _ _ _ _ _ _ _ _ _ _ _ _ _ _ _ _ _] -> w1547
      tunnel: w1546 -> [w1566 w1569 _ w1580 w1587 _ w1600 w1606 w1618 w1621 w1629 w1636 w1641 w1645 _ _ _ _ _ _ _ _ _ _ _ _ _ _ _ _ _ _ _ _ _ _ _ _ _ _ _ _ _]
      tunnel: [_ _ w1572 _ _ _ _ _ _ _ _ _ _ _ _ _ _ _ _ _ _ _ _ _ _ _ _ _ _ _ _ _ _ _ _ _ _ _ _ _ _ _ _] -> w1545
      tunnel: [_ _ _ _ _ _ _ _ _ _ _ _ _ _ _ _ _ _ _ _ _ _ _ _ _ _ _ _ _ TRUE TRUE TRUE TRUE TRUE TRUE TRUE _ _ _ _ _ _ _] -> w1542
      tunnel: [_ _ _ _ _ _ _ _ _ _ _ _ _ _ _ _ _ _ _ _ _ _ _ _ _ _ _ _ _ T5."MAIN" ("Tab Control") T5."PERFORMANCE TEST SETUP" ("Tab Control") T5."AGEING TEST SETUP" ("Tab Control") T5."SYSTEM DATA" ("Tab Control") T5."MFC" ("Tab Control") T5."ANALYSER DATA" ("Tab Control") T5."ALARM LOG" ("Tab Control") _ _ _ _ _ _ _] -> w1541
      tunnel: [_ _ _ _ _ _ _ _ _ _ _ _ _ _ _ _ _ _ _ _ _ _ _ _ _ _ _ _ _ TRUE w1809 w1813 w1817 w1821 w1825 w1829 _ _ _ _ _ _ _] -> w1540
      tunnel: [_ _ _ _ _ _ _ _ _ _ _ _ _ _ _ _ _ _ _ _ _ _ _ _ _ _ _ _ _ w1806 TRUE w1813 w1817 w1821 w1825 w1829 _ _ _ _ _ _ _] -> w1539
      tunnel: [_ _ _ _ _ _ _ _ _ _ _ _ _ _ _ _ _ _ _ _ _ _ _ _ _ _ _ _ _ w1806 w1809 TRUE w1817 w1821 w1825 w1829 _ _ _ _ _ _ _] -> w1538
      tunnel: [_ _ _ _ _ _ _ _ _ _ _ _ _ _ _ _ _ _ _ _ _ _ _ _ _ _ _ _ _ w1806 w1809 w1813 TRUE w1821 w1825 w1829 _ _ _ _ _ _ _] -> w1537
      tunnel: [_ _ _ _ _ _ _ _ _ _ _ _ _ _ _ _ _ _ _ _ _ _ _ _ _ _ _ _ _ w1806 w1809 w1813 w1817 TRUE w1825 w1829 _ _ _ _ _ _ _] -> w1536
      tunnel: [_ _ _ _ _ _ _ _ _ _ _ _ _ _ _ _ _ _ _ _ _ _ _ _ _ _ _ _ _ w1806 w1809 w1813 w1817 w1821 TRUE w1829 _ _ _ _ _ _ _] -> w1535
      tunnel: [_ _ _ _ _ _ _ _ _ _ _ _ _ _ _ _ _ _ _ _ _ _ _ _ _ _ _ _ _ w1806 w1809 w1813 w1817 w1821 w1825 TRUE _ _ _ _ _ _ _] -> w1534
      tunnel: w1519 -> [_ _ _ _ _ _ _ _ _ _ _ _ _ _ _ _ _ _ _ _ _ _ _ _ _ _ _ _ w1803 _ _ _ _ _ _ _ _ _ _ _ _ w1853 _]
      event Timeout {
        n625 = event-data() -> ()  [unwired: 1 in, 2 out]
        n626 = Enqueue Element(queue=w1568, element=Control_3."main" ("Enum")) -> ()  [unwired: 2 in, 3 out]
      }
      event "Clear subcycle": Value Change {
        n627 = event-data() -> ()  [unwired: 1 in, 5 out]
        n628 = Enqueue Element(queue=w1570, element=Control_3."clear table 1" ("Enum")) -> ()  [unwired: 2 in, 3 out]
      }
      event Panel Close? {
        n629 = event-data() -> ()  [unwired: 1 in, 3 out]
        n630 = Two Button Dialog(message="This command will close Eyecat!\nDo you wish to continue?", 1:"No" ("F button name (\"Cancel\")"), 2:"Yes" ("T button name (\"OK\")")) -> (T button?=w1572:bool)
        n631 = Not(x=w1572) -> (.not. x?=w1573:bool)
        n632 = event-data("Discard?"=w1573) -> ()  [unwired: 1 in, 1 out]
      }
      event "Save sCycle": Value Change {
        n633 = event-data() -> ()  [unwired: 1 in, 5 out]
        n634 = local read "Sub-Cycle Pattern"() -> (w1577:string[][])
        n635 = call "Time column check.vi"("Array"=w1577) -> ("Mistake?"=w1578:bool)  [unwired: 10 in]
        n636 = case shown="False" w1578 {
          tunnel: w1579 -> [w1581 _]
          frame False {
            n637 = Enqueue Element(queue=w1581, element=Control_3."save subc") -> (queue out=w1583:refnum<queue>)  [unwired: 2 in, 2 out]
            n638 = Enqueue Element(queue=w1583, element=Control_3."update list 1") -> ()  [unwired: 2 in, 3 out]
          }
          frame True {
            n639 = One Button Dialog(message="The time sequence is incorrect!\nReview and save again!") -> ()  [unwired: 1 in, 1 out]
          }
        }
      }
      event "Load sCycle": Value Change {
        w1586 = FALSE ("Compile Test Button 2")
        n640 = event-data() -> ()  [unwired: 1 in, 5 out]
        n641 = Enqueue Element(queue=w1588, element=Control_3."load subc") -> ()  [unwired: 2 in, 3 out]
        n642 = local write "Test Compiled"(w1586) -> ()
        n643 = local write "Compile Test Button 2"(w1586) -> ()
      }
      event "Export Cycle": Value Change {
        n644 = event-data() -> ()  [unwired: 1 in, 6 out]
        n645 = Equal?(x="Export Cycle", y=TRUE) -> (x = y?=w1591:bool)
        n646 = case shown="True" w1591 {
          tunnel: w1590 -> [_ w1595]
          frame False {
          }
          frame True {
            n647 = Enqueue Element(queue=w1595, element=Control_3."Export Cycle") -> ()  [unwired: 2 in, 3 out]
          }
        }
      }
      event "Delete sCycle": Value Change {
        n648 = event-data() -> ()  [unwired: 1 in, 5 out]
        n649 = Enqueue Element(queue=w1601, element=Control_3."delete subc") -> (queue out=w1603:refnum<queue>)  [unwired: 2 in, 2 out]
        n650 = Enqueue Element(queue=w1603, element=Control_3."update list 1") -> (queue out=w1599:refnum<queue>)  [unwired: 2 in, 2 out]
        n651 = Enqueue Element(queue=w1599, element=Control_3."update Cycle pattern ") -> (queue out=w1596:refnum<queue>)  [unwired: 2 in, 2 out]
        n652 = Enqueue Element(queue=w1596, element=Control_3."Total time calc") -> ()  [unwired: 2 in, 3 out]
      }
      event "Sub-Cycle Pattern": Mouse Down; "Sub-Cycle Pattern": Value Change {
        n653 = event-data() -> ()  [unwired: 1 in, 3 out]
        n654 = property on="Sub-Cycle Pattern" class="Tbl (strict)"() -> ("EditPos"=w1607:T4)  [unwired: 2 in, 2 out]
        n655 = Unbundle By Name(w1607) -> ("Row"=w1609:i32)  [unwired: 1 out]
        n656 = Less?(x=w1609, y=30) -> (x < y?=w1611:bool)
        n657 = case shown="True" w1611 {
          tunnel: w1608 -> [_ w1616]
          frame False {
            n658 = One Button Dialog(message="This table is limited to 30 entries!") -> ()  [unwired: 1 in, 1 out]
          }
          frame True {
            n659 = Enqueue Element(queue=w1616, element=Control_3."convert to num") -> (queue out=w1615:refnum<queue>)  [unwired: 2 in, 2 out]
            n660 = Enqueue Element(queue=w1615, element=Control_3."calc HC CO") -> ()  [unwired: 2 in, 3 out]
          }
        }
        "EditPos Subc" <- w1606
        "Flag1" <- TRUE
      }
      event "Clear Cycle Pattern": Value Change {
        n661 = event-data() -> ()  [unwired: 1 in, 5 out]
        n662 = Enqueue Element(queue=w1619, element=Control_3."clear table 2" ("Enum")) -> ()  [unwired: 2 in, 3 out]
        n663 = local write "Test Compiled"(FALSE ("Test Compiled")) -> ()
      }
      event "Save Cycle": Value Change {
        n664 = event-data() -> ()  [unwired: 1 in, 5 out]
        n665 = Enqueue Element(queue=w1623, element=Control_3."update Cycle pattern ") -> (queue out=w1622:refnum<queue>)  [unwired: 2 in, 2 out]
        n666 = Enqueue Element(queue=w1622, element=Control_3."save cycle") -> (queue out=w1626:refnum<queue>)  [unwired: 2 in, 2 out]
        n667 = Enqueue Element(queue=w1626, element=Control_3."update list 2") -> ()  [unwired: 2 in, 3 out]
      }
      event "Load Cycle": Value Change {
        n668 = event-data() -> ()  [unwired: 1 in, 5 out]
        n669 = Enqueue Element(queue=w1634, element=Control_3."load cycle") -> (queue out=w1632:refnum<queue>)  [unwired: 2 in, 2 out]
        n670 = Enqueue Element(queue=w1632, element=Control_3."update Cycle pattern ") -> (queue out=w1631:refnum<queue>)  [unwired: 2 in, 2 out]
        n671 = local write "Test Compiled"(FALSE ("Test Compiled")) -> ()
        n672 = Enqueue Element(queue=w1631, element=Control_3."Total time calc") -> ()  [unwired: 2 in, 3 out]
      }
      event "Delete Cycle": Value Change {
        n673 = event-data() -> ()  [unwired: 1 in, 5 out]
        n674 = Enqueue Element(queue=w1639, element=Control_3."delete cycle") -> (queue out=w1638:refnum<queue>)  [unwired: 2 in, 2 out]
        n675 = Enqueue Element(queue=w1638, element=Control_3."update list 2") -> ()  [unwired: 2 in, 3 out]
      }
      event Value Change {
        n676 = event-data() -> ()  [unwired: 1 in, 5 out]
        n677 = Enqueue Element(queue=w1642, element=Control_3."Total time calc") -> ()  [unwired: 2 in, 3 out]
      }
      event "Compile Test Button 2": Value Change {
        n678 = event-data() -> ()  [unwired: 1 in, 5 out]
        n679 = case shown="True" "Compile Test Button 2" {
          tunnel: w1646 -> [_ w1650]
          frame False {
          }
          frame True {
            n680 = case shown="True" FALSE {
              tunnel: w1650 -> [w1651 w1655]
              tunnel: [w1651 w1652] -> w1648
              frame False {
              }
              frame True {
                n681 = Enqueue Element(queue=w1655, element=Control_3."save cycle") -> (queue out=w1653:refnum<queue>)  [unwired: 2 in, 2 out]
                n682 = Enqueue Element(queue=w1653, element=Control_3."update list 2") -> (queue out=w1652:refnum<queue>)  [unwired: 2 in, 2 out]
              }
            }
            n683 = Enqueue Element(queue=w1648, element=Control_3."load test array") -> ()  [unwired: 2 in, 3 out]
          }
        }
      }
      event Value Change {
        n684 = event-data() -> ()  [unwired: 1 in, 5 out]
        n685 = Enqueue Element(queue=w1658, element=Control_3."check scycle name") -> ()  [unwired: 2 in, 3 out]
      }
      event Value Change {
        n686 = event-data() -> ()  [unwired: 1 in, 5 out]
        n687 = Enqueue Element(queue=w1659, element=Control_3."check cycle name") -> ()  [unwired: 2 in, 3 out]
      }
      event Value Change {
        n688 = event-data() -> ()  [unwired: 1 in, 5 out]
        n689 = Square(x="Sample Diameter (mm)") -> (x^2=w1668:T2)
        n690 = Compound Arithmetic op=MULTIPLY(w1668, "Sample Length (mm)", "Number of Samples", 3.141592653589793) -> (w1667:T2)
        n691 = Divide(x=w1667, y=4000000.0) -> (x/y=→"Sample Volume (litres)":T2)
      }
      event Value Change {
        # "O2Eq"
        n692 = event-data() -> ()  [unwired: 1 in, 5 out]
        n693 = local write "Inlet LAMBDA"("Inlet LAMBDA") -> ()
        n694 = local write "Inlet O2 (%)"("Inlet O2 (%)") -> ()
        n695 = Decrement(x="Inlet LAMBDA") -> (x-1=w1683:T2)
        n696 = Multiply(x=4.76, y="Inlet LAMBDA") -> (x*y=w1679:T2)
        n697 = Multiply(x=w1683, y=100.0) -> (x*y=w1681:T2)
        n698 = Add(x=0.33, y=w1679) -> (x+y=w1677:T2)
        n699 = Divide(x=w1681, y=w1677) -> (x/y=w1676:T2)
        n700 = Subtract(x="Inlet O2 (%)", y=w1676) -> (x-y=w1674:T2)
        n701 = Multiply(x=w1674, y=2.0) -> (x*y=→"CO Theory (%)":T2)
        n702 = Divide(x=w1674, y=4.5) -> (x/y=→"HC Theory (%)":T2)
      }
      event Value Change {
        n703 = event-data() -> ()  [unwired: 1 in, 5 out]
        n704 = local write "NO ppm Loff"("NO ppm Loff") -> ()
        n705 = local write "NO:CO Ratio"("NO:CO Ratio") -> ()
        n706 = Divide(x="NO ppm Loff", y=T2 10000.0) -> (x/y=w1686:T2)
        n707 = Multiply(x="NO:CO Ratio", y=w1686) -> (x*y=→"CO Theory (%) NO":T2)
      }
      event Value Change {
        n708 = event-data() -> ()  [unwired: 1 in, 5 out]
        n709 = local read "Sample Volume (litres)"() -> (w1691:T7)
        n710 = Equal?(x=w1691, y=0.0) -> (x = y?=w1690:bool)
        n711 = case shown="False" w1690 {
          tunnel: w1691 -> [w1696 _]
          tunnel: "Test Flow Rate(g/s)" -> [w1693 _]
          frame False {
            w1698 = 60.0 ("y")
            n712 = Multiply(x=w1693, y=w1698) -> (x*y=w1700:T2)
            n713 = Divide(x=w1700, y=1.2) -> (x/y=w1695:T2)
            "Vol Flow @ STP (l/min)" <- w1695
            n714 = Multiply(x=w1695, y=w1698) -> (x*y=w1697:T2)
            n715 = Divide(x=w1697, y=w1696) -> (x/y=→"Space Velocity (h-1)":T2)
          }
          frame True {
            n716 = One Button Dialog(message="Review sample specification first!") -> ()  [unwired: 1 in, 1 out]
          }
        }
      }
      event "Leak Test": Value Change {
        n717 = event-data() -> ()  [unwired: 1 in, 5 out]
        n718 = flat-sequence {
          tunnel: w1703 -> [w1706]
          tunnel: [w1706] -> w1702
          tunnel: w1702 -> [w1711]
          frame #0 {
            n719 = local write "Test number"(u16 5) -> ()
            n720 = local write "Enum 1"(u16 3 ("Test number")) -> ()
          }
          frame #1 {
            n721 = Enqueue Element(queue=w1711, element=Control_3."main" ("Enum")) -> (queue out=w1709:refnum<queue>)  [unwired: 2 in, 2 out]
            n722 = Enqueue Element(queue=w1709, element=Control_3."start test" ("Enum")) -> (queue out=w1708:refnum<queue>)  [unwired: 2 in, 2 out]
            n723 = Enqueue Element(queue=w1708, element=Control_3."Leak Test" ("Enum")) -> ()  [unwired: 2 in, 3 out]
          }
        }
      }
      event "Start Test": Value Change {
        n724 = event-data() -> ()  [unwired: 1 in, 6 out]
        n725 = case shown="True" "Start Test" {
          tunnel: w1714 -> [_ w1730]
          frame False {
          }
          frame True {
            n726 = local read "Test Compiled"() -> (w1722:bool)
            n727 = local read "Log Test Data"() -> (w1727:bool)
            n728 = local read "Test number"() -> (w1717:u16)
            n729 = Boolean To (0,1)(Boolean=w1727) -> (0, 1=w1729:i16)
            n730 = Not(x=w1722) -> (.not. x?=w1721:bool)
            n731 = Equal?(x=u16 4 ("y"), y=w1717) -> (x = y?=w1724:bool)
            n732 = Equal To 0?(x=w1729) -> (x = 0?=w1728:bool)
            n733 = Equal?(x=w1717, y=u16 3) -> (x = y?=w1719:bool)
            n734 = And(x=w1721, y=w1724) -> (x .and. y?=w1723:bool)
            n735 = case shown="True" w1728 {
              tunnel: [TRUE ("T button?") w1740] -> w1716
              frame False {
              }
              frame True {
                # "Log Data Check"
                n736 = Two Button Dialog(message="You are not currently logging data!\nDo you wish to continue?", 1:"No" ("T button name (\"OK\")"), 2:"Yes" ("T button name (\"OK\")")) -> (T button?=w1740:bool)
              }
            }
            n737 = case shown="True" w1723 {
              tunnel: [TRUE ("x") FALSE ("x")] -> w1726
              frame False {
              }
              frame True {
                n738 = One Button Dialog(message="Aging Test not CompiledPlease Compile Test Before Starting", button name ("OK")="Ok") -> ()  [unwired: 1 out]
              }
            }
            n739 = case shown="True" w1719 {
              tunnel: [TRUE ("x") TRUE ("x")] -> w1715
              frame False {
              }
              frame True {
                n740 = One Button Dialog(message="Reminder: Please Check that Fresh Lambda Sensors have been Installed", button name ("OK")="Ok") -> ()  [unwired: 1 out]
              }
            }
            n741 = Compound Arithmetic op=AND(w1726, w1715, w1716) -> (w1725:bool)
            n742 = local write "Start Test"(w1725) -> ()
            n743 = case shown="True" w1725 {
              tunnel: w1730 -> [_ w1745]
              frame False {
              }
              frame True {
                n744 = flat-sequence {
                  tunnel: w1745 -> [w1747]
                  tunnel: [w1747] -> w1744
                  tunnel: w1744 -> [w1751]
                  frame #0 {
                    n745 = local write "Enum 1"(u16 1 ("Test number")) -> ()
                  }
                  frame #1 {
                    n746 = Enqueue Element(queue=w1751, element=Control_3."main" ("Enum")) -> (queue out=w1749:refnum<queue>)  [unwired: 2 in, 2 out]
                    n747 = property on="Stop Test" class="Bool (strict)"("DisabledEnum"=T14."Enabled" ("Disabled")) -> ()  [unwired: 2 in, 2 out]
                    n748 = Enqueue Element(queue=w1749, element=Control_3."start test" ("Enum")) -> ()  [unwired: 2 in, 3 out]
                  }
                }
              }
            }
          }
        }
      }
      event "Log Test Data": Value Change {
        n749 = event-data() -> ()  [unwired: 1 in, 6 out]
        n750 = property on="File Name" class="Str (strict)"() -> ("Value"=w1755:T3)  [unwired: 2 in, 2 out]
        n751 = String Length(string=w1755) -> (length=w1754:i32)
        n752 = Equal To 0?(x=w1754) -> (x = 0?=w1753:bool)
        n753 = case shown="True" w1753 {
          frame False {
          }
          frame True {
            n754 = One Button Dialog(message="A filename has not been entered!") -> ()  [unwired: 1 in, 1 out]
          }
        }
      }
      event "Stop Test": Value Change {
        n755 = event-data() -> ()  [unwired: 1 in, 6 out]
        n756 = case shown="True" "Stop Test" {
          tunnel: w1758 -> [_ w1760]
          frame False {
          }
          frame True {
            n757 = flat-sequence {
              tunnel: w1760 -> [w1766]
              tunnel: [w1766] -> w1764
              tunnel: [w1765] -> w1763
              tunnel: w1764 -> [w1770]
              tunnel: [w1769] -> w1762
              tunnel: w1763 -> [w1769]
              tunnel: [w1768] -> w1761
              tunnel: w1762 -> [w1774]
              tunnel: w1761 -> [w1773]
              tunnel: [T14."Disabled and Grayed Out" ("Disabled")] -> _
              frame #0 {
                n758 = local read "Connected?"() -> (w1765:bool)
                n759 = local write "Stop Cmd"(T2 1.0 ("Stop Cmd")) -> ()
              }
              frame #1 {
                n760 = Enqueue Element(queue=w1770, element=Control_3."main" ("Enum")) -> (queue out=w1768:refnum<queue>)  [unwired: 2 in, 2 out]
              }
              frame #2 {
                n761 = case shown="True" w1774 {
                  tunnel: w1773 -> [w1775 w1778]
                  tunnel: [w1775 w1777] -> _
                  frame False {
                  }
                  frame True {
                    n762 = local write "Connected?"(FALSE ("Connected?")) -> ()
                    n763 = Enqueue Element(queue=w1778, element=Control_3."Multigas disconnect" ("Enum")) -> (queue out=w1777:refnum<queue>)  [unwired: 2 in, 2 out]
                  }
                }
              }
            }
            n764 = local write "Start Test"(FALSE ("Start Test")) -> ()
          }
        }
      }
      event "Stopped?": Value Change {
        n765 = event-data() -> ()  [unwired: 1 in, 5 out]
        n766 = flat-sequence {
          tunnel: w1782 -> [w1786]
          tunnel: [w1785] -> w1781
          tunnel: [w1784] -> w1780
          tunnel: w1781 -> [w1788]
          tunnel: w1780 -> [w1787]
          frame #0 {
            n767 = local read "Connected?"() -> (w1784:bool)
            n768 = Enqueue Element(queue=w1786, element=Control_3."main" ("Enum")) -> (queue out=w1785:refnum<queue>)  [unwired: 2 in, 2 out]
          }
          frame #1 {
            n769 = case shown="True" w1787 {
              tunnel: w1788 -> [_ w1789]
              frame False {
              }
              frame True {
                n770 = local write "Connected?"(FALSE ("Connected?")) -> ()
                n771 = Enqueue Element(queue=w1789, element=Control_3."Multigas disconnect" ("Enum")) -> ()  [unwired: 2 in, 3 out]
              }
            }
          }
        }
      }
      event "Alarm ack": Value Change {
        # "system alarm - set to off"
        n772 = event-data() -> ()  [unwired: 1 in, 5 out]
        n773 = local write "Acknowledge"(TRUE ("Acknowledge")) -> ()
        n774 = property on="Soft Alarm" class="Bool (strict)"("Value"=FALSE ("Acknowledge")) -> ()  [unwired: 2 in, 2 out]
        n775 = property on="Alarm ack" class="Bool"("DisabledEnum"=T14."Disabled and Grayed Out" ("Disabled")) -> ()  [unwired: 2 in, 2 out]
      }
      event "Purge System": Value Change {
        n776 = event-data() -> ()  [unwired: 1 in, 5 out]
        n777 = flat-sequence {
          tunnel: w1796 -> [w1798]
          tunnel: [w1798] -> w1795
          tunnel: w1795 -> [w1799]
          frame #0 {
            n778 = local write "Enum 1"(u16 4 ("Test number")) -> ()
          }
          frame #1 {
            n779 = Enqueue Element(queue=w1799, element=Control_3."start test" ("Enum")) -> ()  [unwired: 2 in, 3 out]
          }
        }
      }
      event "Clear log": Value Change {
        n780 = event-data() -> ()  [unwired: 1 in, 5 out]
        n781 = local write "Table"(string[][] [] ("Table")) -> ()
      }
      event "Adv Settings": Value Change {
        # "To be updated"
        # "SO2 conc\nNOx conc\nCO conc\nHC conc\nBleed ratio N2\nBleed ratio CO2"
        n782 = event-data() -> ()  [unwired: 1 in, 6 out]
        n783 = call "Advanced settings MAX.vi"("Admin Path"=w1803) -> ("output cluster"=→"output cluster":T1)
      }
      event "Home 2": Value Change {
        w1806 = FALSE
        n784 = event-data() -> ()  [unwired: 1 in, 6 out]
      }
      event "Performance 2": Value Change {
        w1809 = FALSE
        n785 = event-data() -> ()  [unwired: 1 in, 6 out]
      }
      event "Ageing 2": Value Change {
        w1813 = FALSE
        n786 = event-data() -> ()  [unwired: 1 in, 6 out]
      }
      event "System 2": Value Change {
        w1817 = FALSE
        n787 = event-data() -> ()  [unwired: 1 in, 6 out]
      }
      event "MFC 2": Value Change {
        w1821 = FALSE
        n788 = event-data() -> ()  [unwired: 1 in, 6 out]
      }
      event "Analyser 2": Value Change {
        w1825 = FALSE
        n789 = event-data() -> ()  [unwired: 1 in, 6 out]
      }
      event "Alarm 2": Value Change {
        w1829 = FALSE
        n790 = event-data() -> ()  [unwired: 1 in, 6 out]
      }
      event "Menu": Value Change {
        n791 = event-data() -> ()  [unwired: 1 in, 6 out]
        n792 = case shown="True" "Menu" {
          selector: "Menu" -> [_ w1833]
          frame False {
          }
          frame True {
            n793 = Not(x=w1833) -> (.not. x?=w1834:bool)
            n794 = local write "Back_Menu"(w1834) -> ()
            n795 = control-ref of="Menu_Tab"() -> (w1835:refnum<vi>)
            n796 = call "Move.vi"("Desired Position"=T15 {"Left"=-42, "Top"=-400}, "Obj Ref"=w1835) -> ("New Position"=w1837:T15)  [unwired: 7 in, 2 out]
            n797 = property on="Menu_Tab" class="TabCtl (strict)"("Position"=w1837) -> ()  [unwired: 2 in, 2 out]
          }
        }
      }
      event "Back_Menu": Value Change {
        n798 = event-data() -> ()  [unwired: 1 in, 6 out]
        n799 = case shown="True" "Back_Menu" {
          frame False {
          }
          frame True {
            n800 = control-ref of="Menu_Tab"() -> (w1843:refnum<vi>)
            n801 = local write "Menu"(FALSE ("Menu")) -> ()
            n802 = call "Move.vi"("Sliding Speed (40)"=u32 100, "Desired Position"=T15 {"Left"=-300, "Top"=-412}, "Obj Ref"=w1843) -> ("New Position"=w1841:T15)  [unwired: 6 in, 2 out]
            n803 = property on="Menu_Tab" class="TabCtl (strict)"("Position"=w1841) -> ()  [unwired: 2 in, 2 out]
          }
        }
      }
      event "Import Data": Value Change {
        w1846 = FALSE ("Compile Test Button")
        n804 = event-data() -> ()  [unwired: 1 in, 6 out]
        n805 = case shown="True" "Import Data" {
          tunnel: w1844 -> [_ w1848]
          frame False {
          }
          frame True {
            n806 = Enqueue Element(queue=w1848, element=Control_3."Import Cycle") -> ()  [unwired: 2 in, 3 out]
          }
        }
        n807 = local write "Test Compiled"(w1846) -> ()
        n808 = local write "Compile Test Button 2"(w1846) -> ()
      }
      event "Graph Cycle Box": Value Change {
        n809 = event-data() -> ()  [unwired: 1 in, 6 out]
        n810 = Enqueue Element(queue=w1850, element=Control_3."Display Graph") -> ()  [unwired: 2 in, 3 out]
      }
      event "Graph Cycle Box 2": Value Change {
        n811 = event-data() -> ()  [unwired: 1 in, 6 out]
        n812 = Enqueue Element(queue=w1851, element=Control_3."Display Graph") -> ()  [unwired: 2 in, 3 out]
      }
      event "Admin": Value Change {
        n813 = event-data() -> ()  [unwired: 1 in, 6 out]
        n814 = call "Password.vi"("Admin File Directory"=w1853) -> ()  [unwired: 3 in]
      }
      event "Omicron": Value Change {
        n815 = event-data() -> ()  [unwired: 1 in, 6 out]
        n816 = case shown="False" "Omicron" {
          frame False {
            n817 = flat-sequence {
              tunnel: [u32 13 ("Size:Width")] -> w1856
              tunnel: w1856 -> [w1860]
              tunnel: [T10 [{"String"="CO", "Value"="0"}, {"String"="Air", "Value"="1"}, {"String"="Air Add", "Value"="2"}, {"String"="HC", "Value"="3"}, {"String"="HC Add", "Value"="4"}, {"String"="NO", "Value"="5"}, {"String"="Air Bal", "Value"="6"}, {"String"="HC Bal", "Value"="7"}, {"String"="O2", "Value"="8"}, {"String"="Pre-Cat Valve", "Value"="9"}, {"String"="Bypass", "Value"="10"}, {"String"="Evac", "Value"="11"}] ("Strings And Values []")] -> w1855
              tunnel: w1855 -> [w1866]
              frame #0 {
                n818 = property on="Ageing - Cycle Pattern" class="Tbl (strict)"("Size"=T16 {"Width"=952, "Height"=252}) -> ()  [unwired: 2 in, 2 out]
              }
              frame #1 {
                n819 = for {
                  N: w1860 -> [_]
                  i -> [w1862]
                  n820 = Bundle("Size:Width"=u32 0, w1862) -> (w1864:cluster{"Size:Width":u32, i32})  [unwired: 1 in]
                  n821 = property on="Ageing - Cycle Pattern" class="Tbl (strict)"("Active Cell"=w1864, "Width"=u32 70 ("Size:Width")) -> ()  [unwired: 2 in, 2 out]
                }
                n822 = Decrement(x=w1860) -> (x-1=w1859:u32)
                n823 = property on="Column Length" class="DigNum (strict)"("Value"=w1859) -> ()  [unwired: 2 in, 2 out]
              }
              frame #2 {
                w1869 = 0
                n824 = Bundle(w1869, w1869) -> (w1868:cluster{i32, i32})  [unwired: 1 in]
                n825 = property on="Graph Cycle Box" class="CmbBox"("Strings And Values[]"=w1866) -> ()  [unwired: 2 in, 2 out]
                n826 = property on="Graph Cycle Box 2" class="CmbBox"("Strings And Values[]"=w1866) -> ()  [unwired: 2 in, 2 out]
                n827 = property on="Ageing - Cycle Pattern" class="Tbl (strict)"("Active Cell"=w1868, "Column Headers[]"=string[] ["Index", "CO\nl/min", "Air Main\nl/min", "Air Add\nl/min", "HC Main\nl/min", "HC Add\nl/min", "NO\nl/min", "Air Bal\nl/min", "HC Bal\nl/min", "O2\nl/min", "Pre-Cat\nValve", "Bypass\nValve", "Evac \nValve"] ("Row Header Strings[]")) -> ()  [unwired: 2 in, 2 out]
              }
              frame #3 {
                w1870 = "c:\\Setup Files\\Ageing Cycles\\Omega"
                n828 = property on="Load sCycle" class="Bool"("Position"=T15 {"Left"=1457, "Top"=-119}) -> ()  [unwired: 2 in, 2 out]
                n829 = property on="Clear subcycle" class="Bool"("Position"=T15 {"Left"=1457, "Top"=-57}) -> ()  [unwired: 2 in, 2 out]
                n830 = property on="Export Cycle" class="Bool"("Position"=T15 {"Left"=1459, "Top"=5}) -> ()  [unwired: 2 in, 2 out]
                n831 = String To Path(string=w1870) -> (path=w1879:path)
                n832 = property on="Cycle Directory" class="Str"("Value"=w1870) -> ()  [unwired: 2 in, 2 out]
                n833 = List Folder(path=w1879, pattern="*.eyes") -> (filenames=w1877:string[])  [unwired: 2 in, 3 out]
                n834 = property on="Cycle List" class="LstBox (strict)"("Position"=T15 {"Left"=1013, "Top"=-307}, "Item Names"=w1877) -> ()  [unwired: 2 in, 2 out]
                n835 = property on="Import Data" class="Bool"("Position"=T15 {"Left"=1458, "Top"=-305}) -> ()  [unwired: 2 in, 2 out]
                n836 = property on="Delete sCycle" class="Bool"("Position"=T15 {"Left"=1457, "Top"=-243}) -> ()  [unwired: 2 in, 2 out]
                n837 = property on="Save sCycle" class="Bool"("Position"=T15 {"Left"=1439, "Top"=-181}) -> ()  [unwired: 2 in, 2 out]
              }
              frame #4 {
                n838 = One Button Dialog(message="Machine Updated", button name ("OK")="OK") -> ()  [unwired: 1 out]
              }
            }
          }
          frame True {
            n839 = flat-sequence {
              tunnel: [20 ("Size:Width")] -> w1884
              tunnel: w1884 -> [w1887]
              tunnel: [T10 [{"String"="CO-1", "Value"="0"}, {"String"="Air-1", "Value"="1"}, {"String"="Air-1 Add", "Value"="2"}, {"String"="HC-1", "Value"="3"}, {"String"="HC-1 Add", "Value"="4"}, {"String"="O2-1", "Value"="5"}, {"String"="CO-2", "Value"="6"}, {"String"="Air-2", "Value"="7"}, {"String"="Air-2 Add", "Value"="8"}, {"String"="HC-2", "Value"="9"}, {"String"="HC-2 Add", "Value"="10"}, {"String"="O2-2", "Value"="11"}, {"String"="Air Bal", "Value"="12"}, {"String"="HC Bal", "Value"="13"}, {"String"="Cat-1 Valve", "Value"="14"}, {"String"="Cat-2 Valve", "Value"="15"}, {"String"="Bypass Valve", "Value"="16"}, {"String"="Evac-1", "Value"="17"}, {"String"="Evac-2", "Value"="18"}] ("Strings And Values []")] -> w1883
              tunnel: w1883 -> [w1894]
              frame #0 {
                n840 = property on="Ageing - Cycle Pattern" class="Tbl (strict)"("Size"=T16 {"Width"=1449, "Height"=252}) -> ()  [unwired: 2 in, 2 out]
              }
              frame #1 {
                n841 = Decrement(x=w1887) -> (x-1=w1888:i32)
                n842 = for {
                  N: w1887 -> [_]
                  i -> [w1890]
                  n843 = Bundle("Size:Width"=0, w1890) -> (w1892:cluster{"Size:Width":i32, i32})  [unwired: 1 in]
                  n844 = property on="Ageing - Cycle Pattern" class="Tbl (strict)"("Active Cell"=w1892, "Width"=u32 70 ("Size:Width")) -> ()  [unwired: 2 in, 2 out]
                }
                n845 = property on="Column Length" class="DigNum (strict)"("Value"=w1888) -> ()  [unwired: 2 in, 2 out]
              }
              frame #2 {
                w1897 = 0
                n846 = Bundle(w1897, w1897) -> (w1896:cluster{i32, i32})  [unwired: 1 in]
                n847 = property on="Graph Cycle Box" class="CmbBox"("Strings And Values[]"=w1894) -> ()  [unwired: 2 in, 2 out]
                n848 = property on="Graph Cycle Box 2" class="CmbBox"("Strings And Values[]"=w1894) -> ()  [unwired: 2 in, 2 out]
                n849 = property on="Ageing - Cycle Pattern" class="Tbl (strict)"("Active Cell"=w1896, "Column Headers[]"=string[] ["Index", "CO-1\nl/min", "Air-1 Main\nl/min", "Air-1 Add\nl/min", "HC-1 Main\nl/min", "HC-1 Add\nl/min", "O2-1\nl/min", "CO-2\nl/min", "Air-2 Main\nl/min", "Air-2 Add\nl/min", "HC-2 Main\nl/min", "HC-2 Add\nl/min", "O2-2\nl/min", "Air Bal\nl/min", "HC Bal\nl/min", "Cat-1\nValve", "Cat-2\nValve", "Bypass\nValve", "Evac-1\nValve", "Evac-2\nValve"] ("Row Header Strings[]")) -> ()  [unwired: 2 in, 2 out]
              }
              frame #3 {
                w1898 = "c:\\Setup Files\\Ageing Cycles\\Omicron"
                n850 = property on="Load sCycle" class="Bool"("Position"=T15 {"Left"=1507, "Top"=182}) -> ()  [unwired: 2 in, 2 out]
                n851 = property on="Clear subcycle" class="Bool"("Position"=T15 {"Left"=1507, "Top"=244}) -> ()  [unwired: 2 in, 2 out]
                n852 = property on="Export Cycle" class="Bool"("Position"=T15 {"Left"=1509, "Top"=306}) -> ()  [unwired: 2 in, 2 out]
                n853 = String To Path(string=w1898) -> (path=w1907:path)
                n854 = property on="Cycle Directory" class="Str"("Value"=w1898) -> ()  [unwired: 2 in, 2 out]
                n855 = List Folder(path=w1907, pattern="*.eyes") -> (filenames=w1905:string[])  [unwired: 2 in, 3 out]
                n856 = property on="Cycle List" class="LstBox (strict)"("Position"=T15 {"Left"=1482, "Top"=-307}, "Item Names"=w1905) -> ()  [unwired: 2 in, 2 out]
                n857 = property on="Import Data" class="Bool"("Position"=T15 {"Left"=1508, "Top"=-4}) -> ()  [unwired: 2 in, 2 out]
                n858 = property on="Delete sCycle" class="Bool"("Position"=T15 {"Left"=1507, "Top"=58}) -> ()  [unwired: 2 in, 2 out]
                n859 = property on="Save sCycle" class="Bool"("Position"=T15 {"Left"=1489, "Top"=120}) -> ()  [unwired: 2 in, 2 out]
              }
              frame #4 {
                n860 = One Button Dialog(message="Machine Updated", button name ("OK")="OK") -> ()  [unwired: 1 out]
              }
            }
          }
        }
      }
    }
    "stop 2" <- w1545
    n861 = local write "Tab Control"(w1543) -> ()
    n862 = case shown="False" w1542 {
      tunnel: [w1557 w1565] -> w1544
      tunnel: w1543 -> [w1557 _]
      tunnel: w1541 -> [_ w1565]
      tunnel: w1540 -> [_ w1564]
      tunnel: w1539 -> [_ w1563]
      tunnel: w1538 -> [_ w1562]
      tunnel: w1537 -> [_ w1561]
      tunnel: w1536 -> [_ w1560]
      tunnel: w1535 -> [_ w1559]
      tunnel: w1534 -> [_ w1558]
      tunnel: [w1555 w1564] -> w1533
      tunnel: [w1554 w1563] -> w1532
      tunnel: [w1550 w1562] -> w1531
      tunnel: [w1551 w1561] -> w1530
      tunnel: [w1552 w1560] -> w1529
      tunnel: [w1553 w1559] -> w1528
      tunnel: [w1556 w1558] -> w1527
      tunnel: w1526 -> [w1555 _]
      tunnel: w1525 -> [w1554 _]
      tunnel: w1524 -> [w1556 _]
      tunnel: w1523 -> [w1553 _]
      tunnel: w1522 -> [w1552 _]
      tunnel: w1521 -> [w1551 _]
      tunnel: w1520 -> [w1550 _]
      frame False {
      }
      frame True {
      }
    }
    n863 = local write "MFC 2"(w1529) -> ()
    n864 = local write "Home 2"(w1533) -> ()
    n865 = local write "System 2"(w1530) -> ()
    n866 = local write "Alarm 2"(w1527) -> ()
    n867 = local write "Ageing 2"(w1531) -> ()
    n868 = local write "Analyser 2"(w1528) -> ()
    n869 = local write "Performance 2"(w1532) -> ()
  }
  n870 = node-c288(w59) -> ()  [unwired: 1 out]
  n871 = node-c288(w57) -> ()  [unwired: 1 out]
  n872 = node-c288(w55) -> ()  [unwired: 1 out]
  n873 = node-c288(w53) -> ()  [unwired: 1 out]
  n874 = node-c288(w51) -> ()  [unwired: 1 out]
  n875 = node-c288() -> (w27:T12)  [unwired: 4 in]
  n876 = node-c288(w30) -> (w46:T12)  [unwired: 3 in]
  n877 = node-c288(w30) -> (w35:T12)  [unwired: 3 in]
  n878 = node-c288(w30) -> (w33:T12)  [unwired: 3 in]
  n879 = timed-loop {
    timing: w27 -> [_]
    timing-out: [_] -> w26
    stop <- _ stop-if-true
    n880 = node-c288() -> ()  [unwired: 1 in, 1 out]
    n881 = shared-variable "RT CompactRIO Target\\Library 1.lvlib\\Send Text?"() -> (w1911:bool)  [unwired: 1 in, 1 out]
    n882 = case shown="True" w1911 {
      tunnel: [TRUE w1913] -> _
      frame False {
      }
      frame True {
        n883 = flat-sequence {
          tunnel: [string[] ["+447849454694"] ("phoneNumbers")] -> w1915
          tunnel: ["Alarm in V4!"] -> w1914
          tunnel: w1915 -> [w1919]
          tunnel: w1914 -> [w1918]
          tunnel: [FALSE] -> w1913
          frame #0 {
          }
          frame #1 {
            n884 = call "SMS.vi"("text"=w1918, "phoneNumbers"=w1919) -> ()  [unwired: 10 in]
          }
          frame #2 {
          }
        }
      }
    }
    n885 = node-c288() -> ()  [unwired: 1 in, 1 out]
  }
  n886 = timed-loop {
    timing: w46 -> [_]
    timing-out: [_] -> w45
    tunnel: w31 -> [w1934]
    shift-right: [w1929] -> _
    shift-left: 0 ("length") -> [w1926]
    stop <- _ stop-if-true
    n887 = node-c288() -> ()  [unwired: 1 in, 1 out]
    n888 = call-poly <vilib>:"Read From Spreadsheet File.vi"("file path (dialog if empty)"=w1934) -> ("first row"=w1932:string[])  [unwired: 6 in, 4 out]
    n889 = local read "Mexa-1"() -> (w1928:bool)
    n890 = Index Array(array=w1932, index=0 ("length")) -> (element=w1931:string)
    n891 = case shown="False" w1928 {
      tunnel: w1931 -> [_ w1942]
      tunnel: [FALSE ("Ping Successful?") w1941] -> w1923
      tunnel: [0 ("length") w1940] -> w1925
      tunnel: w1926 -> [_ w1940]
      frame False {
      }
      frame True {
        n892 = call "Ping.vi"("IP address"=w1942) -> ("Ping Successful?"=w1941:bool)  [unwired: 9 in, 1 out]
      }
    }
    "Mexa 1 IP" <- w1923
    n893 = Not(x=w1923) -> (.not. x?=w1924:bool)
    n894 = Equal To 0?(x=w1925) -> (x = 0?=w1927:bool)
    n895 = Compound Arithmetic op=AND(w1924, w1927, w1928) -> (w1930:bool)
    n896 = case shown="True" w1930 {
      tunnel: [w1935 1 ("length")] -> w1929
      tunnel: w1925 -> [w1935 _]
      frame False {
      }
      frame True {
        n897 = One Button Dialog(message="Mexa 1 not found on Network\nPlease Disconnect") -> ()  [unwired: 1 in, 1 out]
      }
    }
    n898 = node-c288() -> ()  [unwired: 1 in, 1 out]
  }
  n899 = timed-loop {
    timing: w35 -> [_]
    timing-out: [_] -> w34
    tunnel: w31 -> [w1956]
    shift-right: [w1951] -> _
    shift-left: 0 ("length") -> [w1948]
    stop <- _ stop-if-true
    n900 = node-c288() -> ()  [unwired: 1 in, 1 out]
    n901 = call-poly <vilib>:"Read From Spreadsheet File.vi"("file path (dialog if empty)"=w1956) -> ("first row"=w1954:string[])  [unwired: 6 in, 4 out]
    n902 = local read "Mexa-2"() -> (w1950:bool)
    n903 = Index Array(array=w1954, index=2 ("length")) -> (element=w1953:string)
    n904 = case shown="False" w1950 {
      tunnel: w1953 -> [_ w1964]
      tunnel: [FALSE ("Ping Successful?") w1963] -> w1945
      tunnel: [0 ("length") w1962] -> w1947
      tunnel: w1948 -> [_ w1962]
      frame False {
      }
      frame True {
        n905 = call "Ping.vi"("IP address"=w1964) -> ("Ping Successful?"=w1963:bool)  [unwired: 9 in, 1 out]
      }
    }
    "Mexa 2 IP" <- w1945
    n906 = Not(x=w1945) -> (.not. x?=w1946:bool)
    n907 = Equal To 0?(x=w1947) -> (x = 0?=w1949:bool)
    n908 = Compound Arithmetic op=AND(w1946, w1949, w1950) -> (w1952:bool)
    n909 = case shown="True" w1952 {
      tunnel: [w1957 1 ("length")] -> w1951
      tunnel: w1947 -> [w1957 _]
      frame False {
      }
      frame True {
        n910 = One Button Dialog(message="Mexa 2 not found on Network\nPlease Disconnect") -> ()  [unwired: 1 in, 1 out]
      }
    }
    n911 = node-c288() -> ()  [unwired: 1 in, 1 out]
  }
  n912 = timed-loop {
    timing: w33 -> [_]
    timing-out: [_] -> w32
    tunnel: w31 -> [w1978]
    shift-right: [w1973] -> _
    shift-left: 0 ("length") -> [w1970]
    stop <- _ stop-if-true
    n913 = node-c288() -> ()  [unwired: 1 in, 1 out]
    n914 = call-poly <vilib>:"Read From Spreadsheet File.vi"("file path (dialog if empty)"=w1978) -> ("first row"=w1976:string[])  [unwired: 6 in, 4 out]
    n915 = local read "Mexa-3"() -> (w1972:bool)
    n916 = Index Array(array=w1976, index=4 ("length")) -> (element=w1975:string)
    n917 = case shown="False" w1972 {
      tunnel: w1975 -> [_ w1986]
      tunnel: [FALSE ("Ping Successful?") w1985] -> w1967
      tunnel: [0 ("length") w1984] -> w1969
      tunnel: w1970 -> [_ w1984]
      frame False {
      }
      frame True {
        n918 = call "Ping.vi"("IP address"=w1986) -> ("Ping Successful?"=w1985:bool)  [unwired: 9 in, 1 out]
      }
    }
    "Mexa 3 IP" <- w1967
    n919 = Not(x=w1967) -> (.not. x?=w1968:bool)
    n920 = Equal To 0?(x=w1969) -> (x = 0?=w1971:bool)
    n921 = Compound Arithmetic op=AND(w1968, w1971, w1972) -> (w1974:bool)
    n922 = case shown="True" w1974 {
      tunnel: [w1979 1 ("length")] -> w1973
      tunnel: w1969 -> [w1979 _]
      frame False {
      }
      frame True {
        n923 = One Button Dialog(message="Mexa 3 not found on Network\nPlease Disconnect") -> ()  [unwired: 1 in, 1 out]
      }
    }
    n924 = node-c288() -> ()  [unwired: 1 in, 1 out]
  }
  n925 = node-c288(w45) -> ()  [unwired: 1 out]
  n926 = node-c288(w34) -> ()  [unwired: 1 out]
  n927 = node-c288(w32) -> ()  [unwired: 1 out]
  n928 = node-c288(w26) -> ()  [unwired: 1 out]
  n929 = node-c288(w22) -> ()  [unwired: 1 out]
  n930 = node-c288(w70) -> ()  [unwired: 1 out]
  n931 = node-c288(w76) -> ()  [unwired: 1 out]
  n932 = local write "stop 2"(w78) -> ()
  "Table" <- string[][] [] ("Table")
